vi "NI_controller.VI"(0 "Motion Settings":T1={"No Motion?"=FALSE, "Motion System"=enum."NI 735x", "Motion Bd ID"=1, "Motion Profile"="SMAC1", "# Axis"=1, "Reverse Z axis?"=TRUE, "SMAC Axis"=0, "scan pair"=enum."y-(x) scan", "RT fps"=6.0, "Steps per mm"=[1000, 1000, 1000, 1000], "Motor Parameters"={"velocity ct/s"=[10000.0, 10000.0, 10000.0, 50000.0], "accel ct/s^2"=[50000.0, 50000.0, 50000.0, 200000.0]}, "One Way Scan"=FALSE, "Reverse One Way Scan"=FALSE, "Global Position (mm)"=[], "Plane"=0, "Distance between\nscan lines (um)"=0.0, "Distance between\nscan planes (um)"=0.0, "number of scan planes"=1, "Total steps in line"=0, "Xtra plane\ndistance  (um)"=100, "Xtra planes "=1, "Add Axis"=FALSE, "overshoot cts"=200, "BKPT Shift"=0, "Scan Start Time (ms)"=0, "ESP VISA"="GPIB::1::INSTR", "3rd Axis"=1, "GL Ref Out"=refnum, "Galil Address"=""} {"3rd Axis" items=["x", "y", "z", "w"]; "Xtra planes" min=1; "Xtra plane\ndistance  (um)" min=0; "Distance between\nscan planes (um)" format="%.2f"; "Distance between\nscan lines (um)" format="%.2f"; "SMAC Axis" items=["None"=0, "Axis 1"=1, "Axis 2"=2, "Axis 3"=3, "Axis 4"=4, "Axis 5"=5, "Axis 6"=6, "Axis 7"=7, "Axis 8"=8, "Vector Space 1"=17, "Vector Space 2"=18, "Vector Space 3"=19, "Vector Space 4"=20]; "Motion Bd ID" min=1 max=32 step=1}, 4 "Initialize":bool=TRUE) -> (5 "Motion Settings Out":T1={"No Motion?"=FALSE, "Motion System"=enum."NI 735x", "Motion Bd ID"=1, "Motion Profile"="SMAC1", "# Axis"=1, "Reverse Z axis?"=TRUE, "SMAC Axis"=0, "scan pair"=enum."y-(x) scan", "RT fps"=6.0, "Steps per mm"=[1000, 1000, 1000, 1000], "Motor Parameters"={"velocity ct/s"=[10000.0, 10000.0, 10000.0, 50000.0], "accel ct/s^2"=[50000.0, 50000.0, 50000.0, 200000.0]}, "One Way Scan"=FALSE, "Reverse One Way Scan"=FALSE, "Global Position (mm)"=[], "Plane"=0, "Distance between\nscan lines (um)"=0.0, "Distance between\nscan planes (um)"=0.0, "number of scan planes"=1, "Total steps in line"=0, "Xtra plane\ndistance  (um)"=100, "Xtra planes "=1, "Add Axis"=FALSE, "overshoot cts"=200, "BKPT Shift"=0, "Scan Start Time (ms)"=0, "ESP VISA"="GPIB::1::INSTR", "3rd Axis"=1, "GL Ref Out"=refnum, "Galil Address"=""} {"3rd Axis" items=["x", "y", "z", "w"]; "Xtra planes" min=1; "Xtra plane\ndistance  (um)" min=0; "Distance between\nscan planes (um)" format="%.2f"; "Distance between\nscan lines (um)" format="%.2f"; "SMAC Axis" items=["None"=0, "Axis 1"=1, "Axis 2"=2, "Axis 3"=3, "Axis 4"=4, "Axis 5"=5, "Axis 6"=6, "Axis 7"=7, "Axis 8"=8, "Vector Space 1"=17, "Vector Space 2"=18, "Vector Space 3"=19, "Vector Space 4"=20]; "Motion Bd ID" min=1 max=32 step=1}, 6 "error out":errorcluster)   [LabVIEW 2022 SP3]
uses:
  -NI_MotionRoutines/MotionParameters.ctl
  -NI_MotionRoutines/MotionSys.ctl
  -MotionRoutines/ScanAxis.ctl
  -MotionRoutines/3rdAxis.ctl
  <vilib>/Motion/FlexMotion/CustomControls/CustomControls.llb/AxisOrVectorSpace To Configure.flx
  <vilib>/Motion/FlexMotion/FunctionsVIs/StartStopMotion.llb/Start Motion (8 axes).flx
  <vilib>/Motion/FlexMotion/FunctionsVIs/StartStopMotion.llb/Stop Motion (8 axes).flx
  -MotionRoutines/MotionGlobals.vi
  <vilib>/Motion/FlexMotion/FunctionsVIs/Trajectory.llb/Load Acceleration/Deceleration.flx
  <vilib>/event_ctls.llb/eventvkey.ctl
  <vilib>/Motion/FlexMotion/CustomControls/CustomControls.llb/Axis # (8 axes).flx
panel:
  in  "Cent All":bool
  in  "Position (mm) (Abs)":dbl format="%.3f"
  in  "Axis Tune":enum32{"Axis 1", "Axis 2", "Axis 3", "Axis 4"}(radio)
  in  "Inc. Step\nSize (mm)":dbl=0.5
  out "Found Center":bool
  in  "Cent X":bool
  in  "Cent Y":bool
  in  "Cent Z":bool
  in  "Abs W Pos (mm)":dbl format="%.3f"
  in  "Abs Z Pos (mm)":dbl format="%.3f"
  in  "Abs Y Pos (mm)":dbl format="%.3f"
  in  "Abs X Pos (mm)":dbl format="%.3f"
  in  "Def Abs":bool
  in  "Select V&A":bool
  in  "Slave Axis":u16(ring)=2 items=["Axis 1"=1, "Axis 2"=2, "Axis 3"=3, "Axis 4"=4]
  in  "Master Axis":u16(ring)=1 items=["Axis 1"=1, "Axis 2"=2, "Axis 3"=3, "Axis 4"=4]
  in  "Enable Gearing":bool
  out "Angle":dbl=45.000038009906035
  in  "Ratio Denom":u16=1 min=1 max=32767
  in  "Ratio Num":i16 min=0
  in  "Cent W":bool
  in  "W Position (mm)":dbl format="%.3f"
  in  "FineMi4":bool
  in  "FinePl4":bool
  in  "Rst4":bool
  in  "Ax4Plus":bool
  in  "Ax4Minus":bool
  in  "Z Position (mm)":dbl format="%.3f"
  in  "FineMi3":bool
  in  "FinePl3":bool
  in  "Rst3":bool
  in  "Ax3Plus":bool
  in  "Ax3Minus":bool
  in  "Y Position (mm)":dbl format="%.3f"
  in  "FineMi2":bool
  in  "FinePl2":bool
  in  "Rst2":bool
  in  "Ax2Plus":bool
  in  "Ax2Minus":bool
  in  "X Position (mm)":dbl format="%.3f"
  in  "stop":bool
  in  "FineMi1":bool
  in  "FinePl1":bool
  in  "Rst1":bool
  in  "Ax1Plus":bool
  in  "Ax1Minus":bool
  # "Units are in mm. \"Rst\" zeros the position. Blue circles move 1 cm for linear."
  # "Redefine\nAbs Position"
  # "Be very careful with this mode it is not fully programmed"
  # "X Axis (mm)"
  # "Y Axis  (mm)"
  # "Z Axis (mm)"
  # "LinInd (mm)"
  # "1-D and 2-D B scan settings"
  # "1-D and 2-D B scan settings"
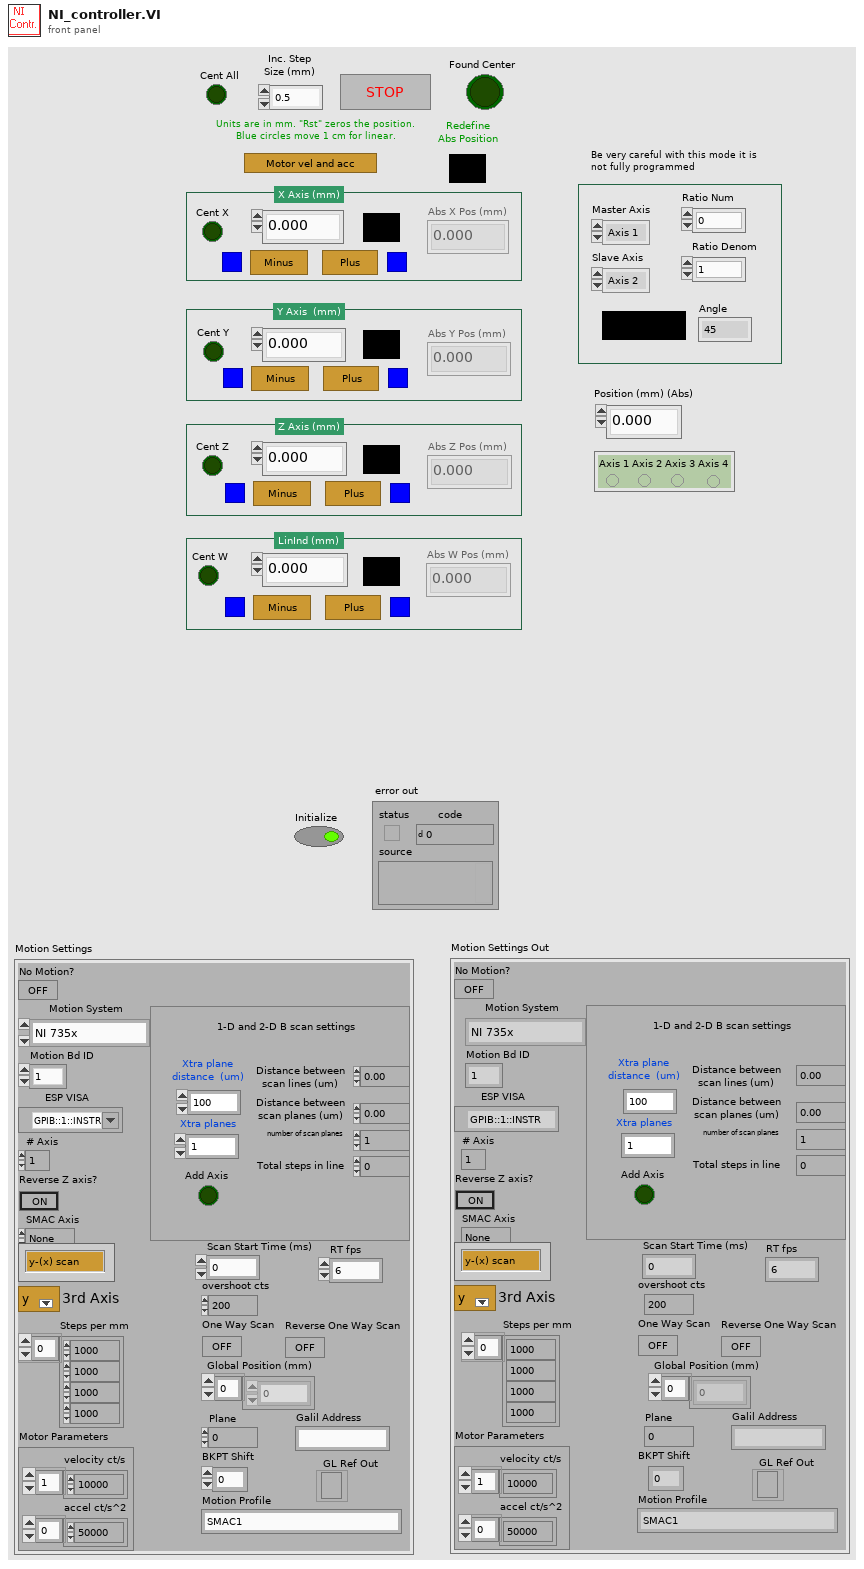
[diagram p1: front panel]
types:
  T1 = typedef "MotionParameters.ctl" = cluster{"No Motion?":bool, "Motion System":T2, "Motion Bd ID":u8, "Motion Profile":string, "# Axis":i8, "Reverse Z axis?":bool, "SMAC Axis":u16, "scan pair":T3, "RT fps":sgl, "Steps per mm":i32[], "Motor Parameters":cluster{"velocity ct/s":dbl[], "accel ct/s^2":dbl[]}, "One Way Scan":bool, "Reverse One Way Scan":bool, "Global Position (mm)":dbl[], "Plane":i32, "Distance between\nscan lines (um)":sgl, "Distance between\nscan planes (um)":sgl, "number of scan planes":i32, "Total steps in line":i32, "Xtra plane\ndistance  (um)":i32, "Xtra planes ":i32, "Add Axis":bool, "overshoot cts":i32, "BKPT Shift":i32, "Scan Start Time (ms)":u32, "ESP VISA":refnum<visa-resource-name>, "3rd Axis":T4, "GL Ref Out":refnum<k7>, "Galil Address":string}
  T2 = typedef "MotionSys.ctl" = enum16{"MM3000", "NI 735x", "Newport ESP", "No Motion Card", "Galil"}
  T3 = typedef "ScanAxis.ctl" = enum16{"y-(x) scan", "x-(y) scan", "z-(x) scan", "z-(y) scan", "y-(z) scan", "x-(z) scan", "w-(x) scan", "w-(y) scan", "w-(z) scan", "x-(w) scan", "y-(w) scan", "z-(w) scan"}
  T4 = typedef "3rdAxis.ctl" = u16
  T5 = enum16{"Absolute Position", "Relative Position", "Velocity", "Relative to Cap Pos", "Modulus Position", "Absolute Contouring", "Relative Contouring"}
  T6 = enum16{"Home", "Index", "Center", "Forward Limit", "Reverse Limit", "Run Sequence"}
  T7 = typedef "Axis # (8 axes).flx" = cluster{"1":bool, "2":bool, "3":bool, "4":bool, "5":bool, "6":bool, "7":bool, "8":bool}
  T8 = enum8{"Enabled", "Disabled", "Disabled and Grayed Out"}
  T9 = typedef "Bd Id Out" = u8
  T10 = typedef "location.ctl" = enum16{"Automatic", "WCM Main", "Hawaii", "Columbia MM3000", "Columbia  NI System", "NYU", "RRI 2", "UHI Allen", "CUMC RT", "Chiba", "Stony Brook", "WCM Microscopy", "WCM Aeoretch", "WCM Optics Lab", "WCM Main 2Axis", "WCM Rotation", "WCM SAM SMAC", "SERI GP"}
  T11 = typedef "AxisOrVectorSpace To Configure.flx" = u16
  T12 = cluster{"Steps per mm[0]":i32, "Steps per mm[1]":i32, "Steps per mm[2]":i32, "Steps per mm[3]":i32}
  T13 = typedef "Resource Out (Enum).flx" = u16
  T14 = typedef "eventvkey.ctl" = enum16{"ASCII", "Enter", "Return", "Shift", "Ctrl", "Alt", "Cmd", "Opt", "Caps", "NumLock", "Clear", "Break", "Up", "Down", "Left", "Right", "Insert", "Delete", "Home", "End", "PageUp", "PageDown", "Escape", "Help", "Pause", "ScrollLock", "F1", "F2", "F3", "F4", "F5", "F6", "F7", "F8", "F9", "F10", "F11", "F12", "F13", "F14", "F15", "F16", "F17", "F18", "F19", "F20", "F21", "F22", "F23", "F24", "Play", "VolumeUp", "VolumeDown", "Mute", "Two Byte Char"}
  T15 = cluster{"Shift":bool, "Ctrl":bool, "Alt":bool, "Cmd":bool, "Opt":bool}
  T16 = typedef "AxisOrVectorSpaceControl To Control.flx" = u16
  T17 = cluster{"Axis/VS Map (Disabled)[0]":bool, "Axis/VS Map (Disabled)[1]":bool, "Axis/VS Map (Disabled)[2]":bool, "Axis/VS Map (Disabled)[3]":bool, "Axis/VS Map (Disabled)[4]":bool, "Axis/VS Map (Disabled)[5]":bool, "Axis/VS Map (Disabled)[6]":bool, "Axis/VS Map (Disabled)[7]":bool, "Axis/VS Map (Disabled)[8]":bool}
  T18 = cluster{"Axis/VS Map (Disabled)[1]":bool, "Axis/VS Map (Disabled)[2]":bool, "Axis/VS Map (Disabled)[3]":bool, "Axis/VS Map (Disabled)[4]":bool, "Axis/VS Map (Disabled)[5]":bool, "Axis/VS Map (Disabled)[6]":bool, "Axis/VS Map (Disabled)[7]":bool, "Axis/VS Map (Disabled)[8]":bool}
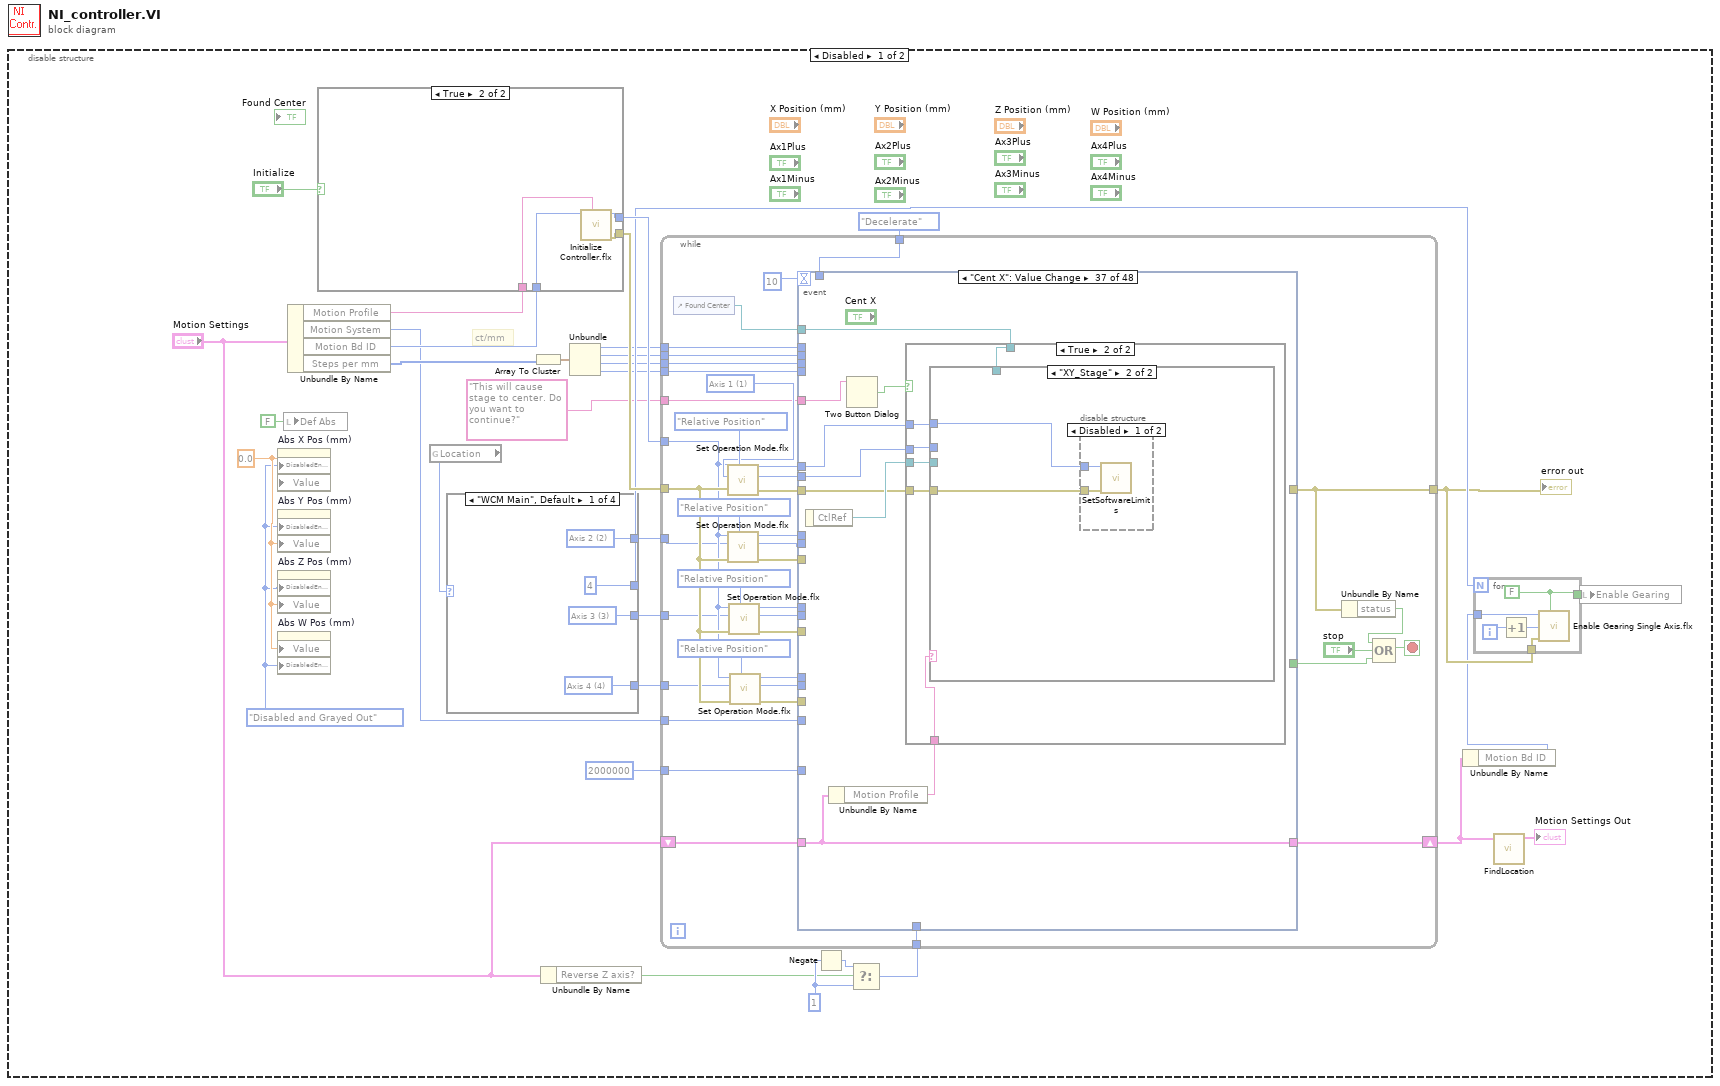
[diagram p0: block diagram]
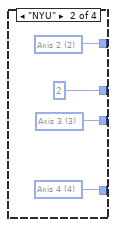
[diagram p2: hidden frame]
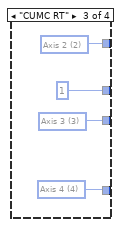
[diagram p3: hidden frame]
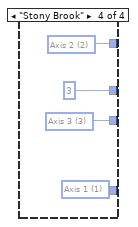
[diagram p4: hidden frame]
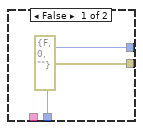
[diagram p5: hidden frame]
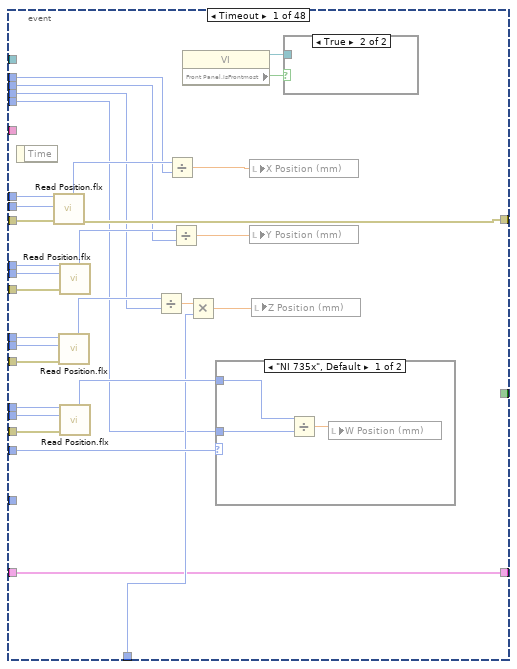
[diagram p6: hidden frame]
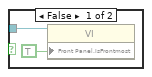
[diagram p7: hidden frame]
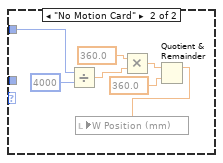
[diagram p8: hidden frame]
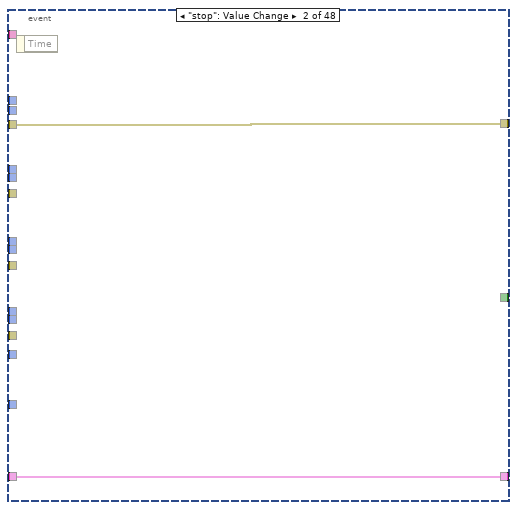
[diagram p9: hidden frame]
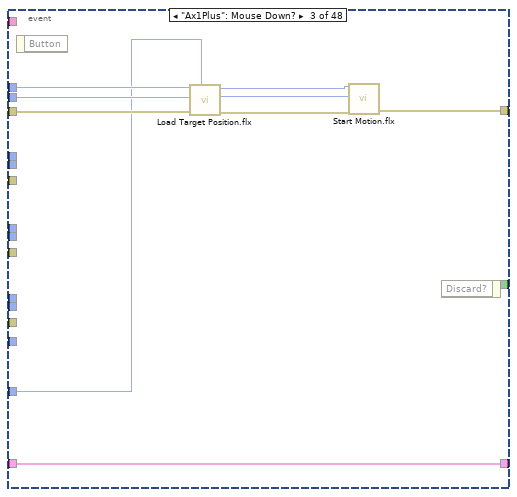
[diagram p10: hidden frame]
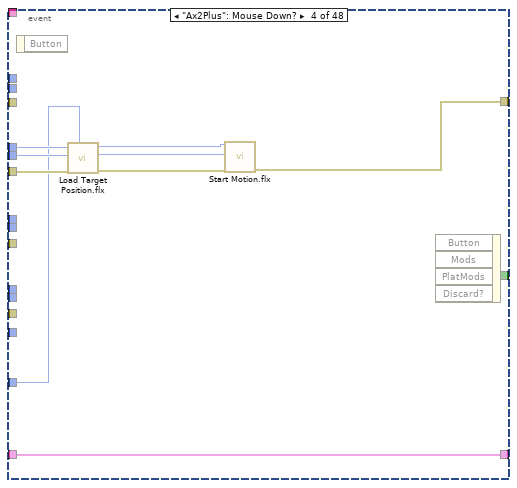
[diagram p11: hidden frame]
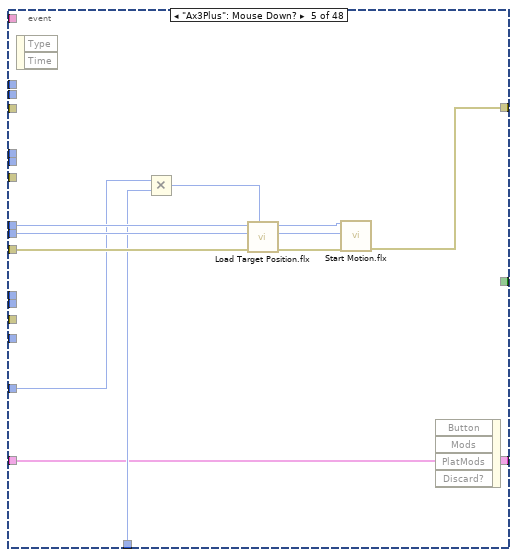
[diagram p12: hidden frame]
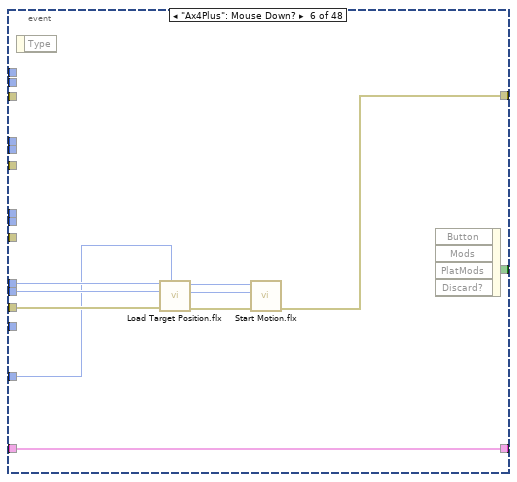
[diagram p13: hidden frame]
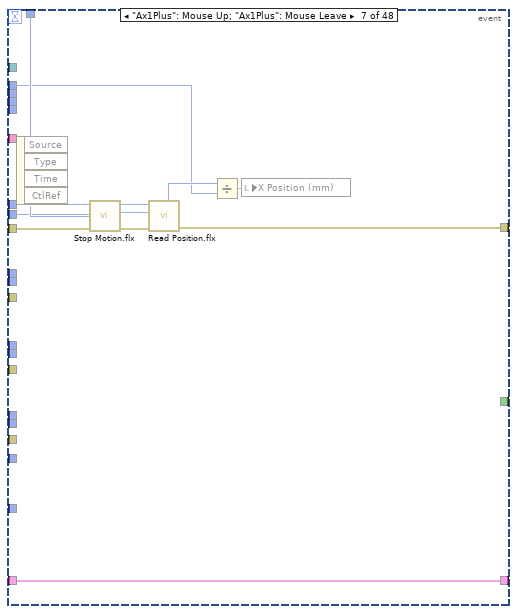
[diagram p14: hidden frame]
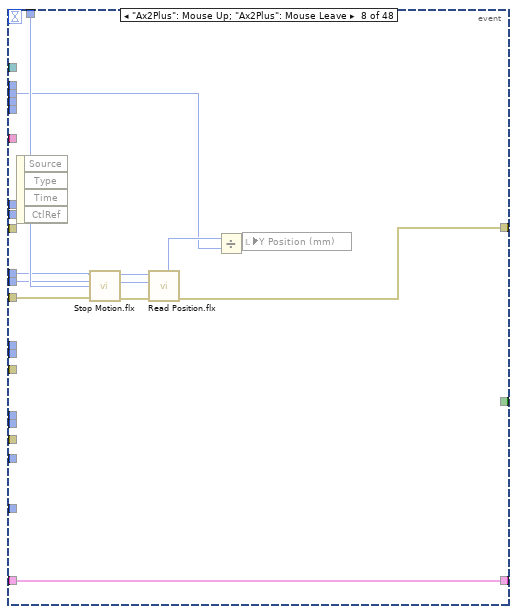
[diagram p15: hidden frame]
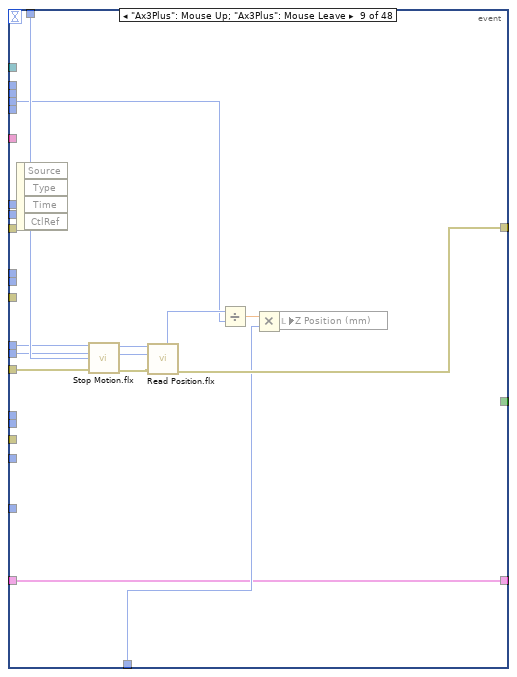
[diagram p16: hidden frame]
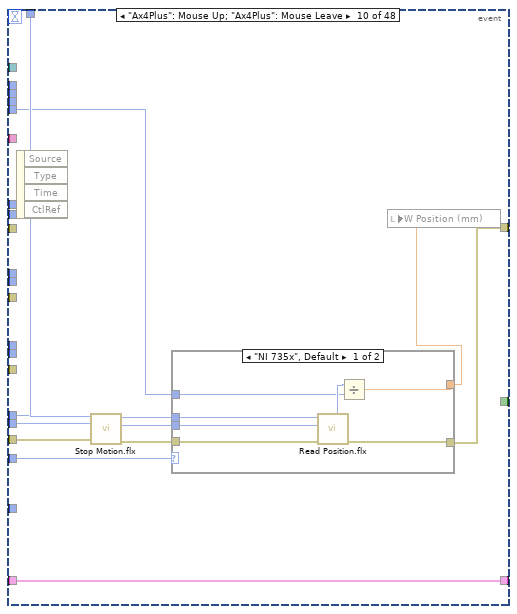
[diagram p17: hidden frame]
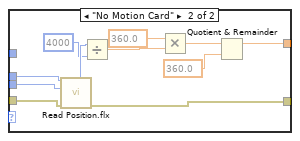
[diagram p18: hidden frame]
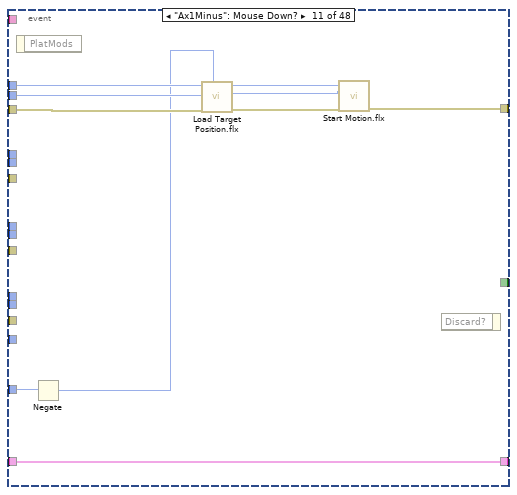
[diagram p19: hidden frame]
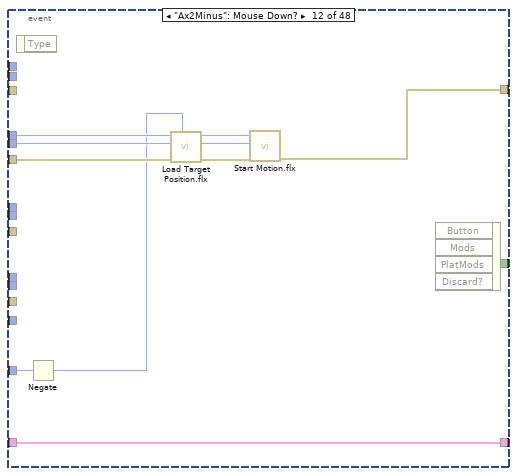
[diagram p20: hidden frame]
diagram:
  n1 = disable-structure shown="Disabled" {
    frame Disabled {
      w5 = T8."Disabled and Grayed Out" ("Disabled")
      w14 = 0.0 ("Abs X Pos (mm)")
      w28 = 1
      # "ct/mm"
      n2 = property on="Abs X Pos (mm)" class="DigNum (strict)"("DisabledEnum"=w5, "Value"=w14) -> ()  [unwired: 2 in, 2 out]
      n3 = property on="Abs Y Pos (mm)" class="DigNum (strict)"("DisabledEnum"=w5, "Value"=w14) -> ()  [unwired: 2 in, 2 out]
      n4 = property on="Abs Z Pos (mm)" class="DigNum (strict)"("DisabledEnum"=w5, "Value"=w14) -> ()  [unwired: 2 in, 2 out]
      n5 = property on="Abs W Pos (mm)" class="DigNum (strict)"("Value"=w14, "DisabledEnum"=w5) -> ()  [unwired: 2 in, 2 out]
      n6 = local write "Def Abs"(FALSE ("Visible")) -> ()
      n7 = Unbundle By Name("Motion Settings") -> ("Motion Profile"=w2:string, "Motion System"=w7:T2, "Motion Bd ID"=w13:u8, "Steps per mm"=w11:i32[])
      n8 = case shown="True" "Initialize" {
        tunnel: [w56 w60] -> w33
        tunnel: [errorcluster {"status"=FALSE, "code"=0, "source"=""} ("error out") w59] -> w32
        tunnel: w13 -> [w56 w58]
        tunnel: w2 -> [_ w57]
        frame False {
        }
        frame True {
          n9 = call <vilib>:"Initialize Controller.flx"("Settings Name"=w57, "Board ID"=w58) -> ("error out"=w59:errorcluster, "Bd ID Out"=w60:T9)  [unwired: 1 in, 5 out]
        }
      }
      n10 = global read "MotionGlobals.vi" "Location"() -> (w22:T10)
      n11 = case shown="\"WCM Main\", Default" w22 {
        tunnel: [w37 w40 w44 w48] -> w25
        tunnel: [w36 w41 w45 w49] -> w24
        tunnel: [4 2 1 3] -> w23
        tunnel: [w34 w38 w42 w46] -> w21
        frame "WCM Main", Default {
          w34 = T11 2 items=["Axis Control"=0, "Axis 1"=1, "Axis 2"=2, "Axis 3"=3, "Axis 4"=4, "Axis 5"=5, "Axis 6"=6, "Axis 7"=7, "Axis 8"=8, "Vector Space Control"=16, "Vector Space 1"=17, "Vector Space 2"=18, "Vector Space 3"=19, "Vector Space 4"=20] ("Axis or Vector Space")
          w37 = T11 4 items=["Axis Control"=0, "Axis 1"=1, "Axis 2"=2, "Axis 3"=3, "Axis 4"=4, "Axis 5"=5, "Axis 6"=6, "Axis 7"=7, "Axis 8"=8, "Vector Space Control"=16, "Vector Space 1"=17, "Vector Space 2"=18, "Vector Space 3"=19, "Vector Space 4"=20] ("Axis or Vector Space")
          w36 = T11 3 items=["Axis Control"=0, "Axis 1"=1, "Axis 2"=2, "Axis 3"=3, "Axis 4"=4, "Axis 5"=5, "Axis 6"=6, "Axis 7"=7, "Axis 8"=8, "Vector Space Control"=16, "Vector Space 1"=17, "Vector Space 2"=18, "Vector Space 3"=19, "Vector Space 4"=20] ("Axis or Vector Space")
        }
        frame "NYU" {
          w38 = T11 2 items=["Axis Control"=0, "Axis 1"=1, "Axis 2"=2, "Axis 3"=3, "Axis 4"=4, "Axis 5"=5, "Axis 6"=6, "Axis 7"=7, "Axis 8"=8, "Vector Space Control"=16, "Vector Space 1"=17, "Vector Space 2"=18, "Vector Space 3"=19, "Vector Space 4"=20] ("Axis or Vector Space")
          w40 = T11 4 items=["Axis Control"=0, "Axis 1"=1, "Axis 2"=2, "Axis 3"=3, "Axis 4"=4, "Axis 5"=5, "Axis 6"=6, "Axis 7"=7, "Axis 8"=8, "Vector Space Control"=16, "Vector Space 1"=17, "Vector Space 2"=18, "Vector Space 3"=19, "Vector Space 4"=20] ("Axis or Vector Space")
          w41 = T11 3 items=["Axis Control"=0, "Axis 1"=1, "Axis 2"=2, "Axis 3"=3, "Axis 4"=4, "Axis 5"=5, "Axis 6"=6, "Axis 7"=7, "Axis 8"=8, "Vector Space Control"=16, "Vector Space 1"=17, "Vector Space 2"=18, "Vector Space 3"=19, "Vector Space 4"=20] ("Axis or Vector Space")
        }
        frame "CUMC RT" {
          w42 = T11 2 items=["Axis Control"=0, "Axis 1"=1, "Axis 2"=2, "Axis 3"=3, "Axis 4"=4, "Axis 5"=5, "Axis 6"=6, "Axis 7"=7, "Axis 8"=8, "Vector Space Control"=16, "Vector Space 1"=17, "Vector Space 2"=18, "Vector Space 3"=19, "Vector Space 4"=20] ("Axis or Vector Space")
          w44 = T11 4 items=["Axis Control"=0, "Axis 1"=1, "Axis 2"=2, "Axis 3"=3, "Axis 4"=4, "Axis 5"=5, "Axis 6"=6, "Axis 7"=7, "Axis 8"=8, "Vector Space Control"=16, "Vector Space 1"=17, "Vector Space 2"=18, "Vector Space 3"=19, "Vector Space 4"=20] ("Axis or Vector Space")
          w45 = T11 3 items=["Axis Control"=0, "Axis 1"=1, "Axis 2"=2, "Axis 3"=3, "Axis 4"=4, "Axis 5"=5, "Axis 6"=6, "Axis 7"=7, "Axis 8"=8, "Vector Space Control"=16, "Vector Space 1"=17, "Vector Space 2"=18, "Vector Space 3"=19, "Vector Space 4"=20] ("Axis or Vector Space")
        }
        frame "Stony Brook" {
          w46 = T11 2 items=["Axis Control"=0, "Axis 1"=1, "Axis 2"=2, "Axis 3"=3, "Axis 4"=4, "Axis 5"=5, "Axis 6"=6, "Axis 7"=7, "Axis 8"=8, "Vector Space Control"=16, "Vector Space 1"=17, "Vector Space 2"=18, "Vector Space 3"=19, "Vector Space 4"=20] ("Axis or Vector Space")
          w48 = T11 1 items=["Axis Control"=0, "Axis 1"=1, "Axis 2"=2, "Axis 3"=3, "Axis 4"=4, "Axis 5"=5, "Axis 6"=6, "Axis 7"=7, "Axis 8"=8, "Vector Space Control"=16, "Vector Space 1"=17, "Vector Space 2"=18, "Vector Space 3"=19, "Vector Space 4"=20] ("Axis or Vector Space")
          w49 = T11 3 items=["Axis Control"=0, "Axis 1"=1, "Axis 2"=2, "Axis 3"=3, "Axis 4"=4, "Axis 5"=5, "Axis 6"=6, "Axis 7"=7, "Axis 8"=8, "Vector Space Control"=16, "Vector Space 1"=17, "Vector Space 2"=18, "Vector Space 3"=19, "Vector Space 4"=20] ("Axis or Vector Space")
        }
      }
      n12 = Array To Cluster(array=w11) -> (cluster=w20:T12)
      n13 = Unbundle By Name("Motion Settings") -> ("Reverse Z axis?"=w12:bool)
      n14 = Unbundle(w20) -> ("Steps per mm[0]"=w19:i32, "Steps per mm[1]"=w18:i32, "Steps per mm[2]"=w17:i32, "Steps per mm[3]"=w16:i32)
      n15 = Negate(x=w28) -> (-x=w30:i32)
      n16 = Select(t=w30, s=w12, f=w28) -> (s? t:f=w29:i32)
      n17 = while {
        tunnel: [w76] -> w9
        tunnel: w32 -> [w89]
        tunnel: w33 -> [w81]
        tunnel: w29 -> [w78]
        tunnel: w7 -> [w77]
        tunnel: 2000000 -> [w75]
        tunnel: enum16{"Decelerate", "Halt", "Kill"}."Decelerate" ("Stop Type (Decel)") -> [w74]
        tunnel: w25 -> [w73]
        tunnel: w24 -> [w72]
        tunnel: w21 -> [w71]
        tunnel: w19 -> [w70]
        tunnel: w18 -> [w69]
        tunnel: w17 -> [w68]
        tunnel: w16 -> [w67]
        shift-right: [w65] -> w4
        shift-left: "Motion Settings" -> [w66]
        tunnel: "This will cause stage to center. Do you want to continue?" ("message") -> [w61]
        stop <- w99 stop-if-true
        w94 = T11 1 items=["Axis Control"=0, "Axis 1"=1, "Axis 2"=2, "Axis 3"=3, "Axis 4"=4, "Axis 5"=5, "Axis 6"=6, "Axis 7"=7, "Axis 8"=8, "Vector Space Control"=16, "Vector Space 1"=17, "Vector Space 2"=18, "Vector Space 3"=19, "Vector Space 4"=20] ("Axis or Vector Space")
        n18 = control-ref of="Found Center"() -> (w63:refnum<vi>)
        n19 = call <vilib>:"Set Operation Mode.flx"("Position Mode (Absolute)"=T5."Relative Position", "error in (no error)"=w89, "Axis or Vector Space"=w94, "Board ID"=w81) -> ("error out"=w96:errorcluster, "Resource Output"=w93:T13, "Bd ID Out"=w97:T9)  [unwired: 2 out]
        n20 = call <vilib>:"Set Operation Mode.flx"("Position Mode (Absolute)"=T5."Relative Position", "error in (no error)"=w89, "Axis or Vector Space"=w71, "Board ID"=w81) -> ("error out"=w88:errorcluster, "Resource Output"=w80:T13, "Bd ID Out"=w79:T9)  [unwired: 2 out]
        n21 = call <vilib>:"Set Operation Mode.flx"("Position Mode (Absolute)"=T5."Relative Position", "error in (no error)"=w89, "Axis or Vector Space"=w72, "Board ID"=w81) -> ("error out"=w85:errorcluster, "Resource Output"=w86:T13, "Bd ID Out"=w87:T9)  [unwired: 2 out]
        n22 = call <vilib>:"Set Operation Mode.flx"("Position Mode (Absolute)"=T5."Relative Position", "error in (no error)"=w89, "Axis or Vector Space"=w73, "Board ID"=w81) -> ("error out"=w82:errorcluster, "Resource Output"=w83:T13, "Bd ID Out"=w84:T9)  [unwired: 2 out]
        n23 = event shown="[36] \"Cent X\": Value Change" {
          selector: _ -> [_ _ _ _ _ _ _ _ _ _ _ _ _ _ _ _ _ _ _ _ _ _ _ _ _ _ _ _ _ _ _ _ _ _ _ _ _ _ _ _ _ _ _ _ _ _ _ _]
          dyn-events: _ -> [_ _ _ _ _ _ _ _ _ _ _ _ _ _ _ _ _ _ _ _ _ _ _ _ _ _ _ _ _ _ _ _ _ _ _ _ _ _ _ _ _ _ _ _ _ _ _ _]
          timeout: 10 -> [_ _ _ _ _ _ _ _ _ _ _ _ _ _ _ _ _ _ _ _ _ _ _ _ _ _ _ _ _ _ _ _ _ _ _ _ _ _ _ _ _ _ _ _ _ _ _ _]
          tunnel: w97 -> [w130 _ w153 _ _ _ w194 _ _ _ w260 _ _ _ w303 _ _ _ w366 _ _ _ w391 _ _ _ w447 _ _ _ w513 _ _ _ _ _ w646 _ _ _ _ _ _ _ w824 _ _ _]
          tunnel: w96 -> [w129 w144 w151 _ _ _ w193 _ _ _ w258 _ _ _ w302 _ _ _ w365 _ _ _ w390 _ _ _ w446 _ _ _ w512 _ _ _ _ _ w650 _ _ _ _ _ _ _ _ _ _ _]
          tunnel: w74 -> [_ _ _ _ _ _ w192 w202 w216 w232 _ _ _ _ w304 w312 w326 w339 _ _ _ _ _ _ _ _ _ _ _ _ _ _ _ _ _ _ _ _ _ _ _ _ _ _ _ _ _ _]
          tunnel: w93 -> [w106 _ w152 _ _ _ w186 _ _ _ w259 _ _ _ w295 _ _ _ w364 _ _ _ w388 _ _ _ w444 _ _ _ w499 _ _ _ _ _ w645 _ _ _ _ _ _ _ w823 _ _ _]
          tunnel: w79 -> [w125 _ _ w159 _ _ _ w201 _ _ _ w267 _ _ _ w311 _ _ _ w372 _ _ _ w401 _ _ _ w457 _ _ _ w520 _ _ _ _ _ w688 _ _ _ w800 w811 _ _ w830 _ _]
          tunnel: w80 -> [w115 _ _ w158 _ _ _ w200 _ _ _ w266 _ _ _ w310 _ _ _ w371 _ _ _ w400 _ _ _ w456 _ _ _ w518 _ _ _ _ _ w687 _ _ _ _ _ _ _ w829 _ _]
          tunnel: w88 -> [w124 _ _ w157 _ _ _ w199 _ _ _ w265 _ _ _ w309 _ _ _ w370 _ _ _ w399 _ _ _ w455 _ _ _ w519 _ _ _ _ _ w685 _ _ _ _ _ _ _ _ _ _]
          tunnel: w87 -> [w123 _ _ _ w170 _ _ _ w215 _ _ _ w279 _ _ _ w325 _ _ _ w378 _ _ _ w413 _ _ _ w469 _ _ _ w538 _ _ _ _ _ w721 _ _ _ _ _ _ _ w838 _]
          tunnel: w86 -> [w122 _ _ _ w169 _ _ _ w214 _ _ _ w278 _ _ _ w324 _ _ _ w377 _ _ _ w412 _ _ _ w468 _ _ _ w537 _ _ _ _ _ w720 _ _ _ _ _ _ _ w837 _]
          tunnel: w85 -> [w121 _ _ _ w168 _ _ _ w213 _ _ _ w277 _ _ _ w323 _ _ _ w376 _ _ _ w411 _ _ _ w467 _ _ _ w536 _ _ _ _ _ w718 _ _ _ _ _ _ _ _ _]
          tunnel: w84 -> [w120 _ _ _ _ w179 _ _ _ w231 _ _ _ w289 _ _ _ w338 _ _ _ w384 _ _ _ w424 _ _ _ w480 _ _ _ w557 w588 _ _ _ _ w757 w763 _ _ _ _ _ _ w844]
          tunnel: w83 -> [w119 _ _ _ _ w178 _ _ _ w230 _ _ _ w288 _ _ _ w337 _ _ _ w383 _ _ _ w423 _ _ _ w479 _ _ _ w556 _ _ _ _ _ w756 _ _ _ _ _ _ _ w843]
          tunnel: w82 -> [w118 _ _ _ _ w177 _ _ _ w229 _ _ _ w287 _ _ _ w336 _ _ _ w382 _ _ _ w422 _ _ _ w478 _ _ _ w555 w589 _ _ _ _ w747 w762 _ _ _ _ _ _ _]
          tunnel: [w112 w144 w147 w156 w165 w176 w185 w197 w212 w223 w254 w264 w273 w286 w296 w307 w322 w333 w362 w368 w374 _ w389 w398 w408 w421 w445 w454 w464 w477 w500 w516 w534 w552 w586 _ _ _ _ _ _ _ _ _ _ _ _ _] -> w76
          tunnel: [_ _ _ _ _ _ _ _ _ _ _ _ _ _ _ _ _ _ _ _ _ w381 _ _ _ _ _ _ _ _ _ _ _ _ _ _ _ _ _ _ _ _ _ _ _ _ _ _] -> _
          tunnel: w78 -> [w109 _ _ _ w167 _ _ _ w209 _ _ _ w276 _ _ _ w319 _ _ _ _ _ _ _ w410 _ _ _ w466 _ _ _ w533 _ _ _ _ _ _ _ _ _ _ _ _ _ w833 _]
          tunnel: w77 -> [w113 _ _ _ _ _ _ _ _ w224 _ _ _ _ _ _ _ w334 _ _ _ _ _ _ _ w420 _ _ _ w476 _ _ _ w551 _ _ _ _ _ _ _ _ _ _ _ _ _ _]
          tunnel: w75 -> [_ _ w146 w155 w164 w175 _ _ _ _ w253 w263 w272 w285 _ _ _ _ _ _ _ _ _ _ _ _ _ _ _ _ _ _ _ _ _ _ _ _ _ _ _ _ _ _ _ _ _ _]
          tunnel: w70 -> [w105 _ _ _ _ _ w184 _ _ _ _ _ _ _ w294 _ _ _ _ _ _ _ w386 _ _ _ w442 _ _ _ w498 _ _ _ _ _ _ _ _ _ _ _ _ _ w822 _ _ _]
          tunnel: w69 -> [w104 _ _ _ _ _ _ w196 _ _ _ _ _ _ _ w306 _ _ _ _ _ _ _ w397 _ _ _ w453 _ _ _ w515 _ _ _ _ _ _ _ _ _ _ _ _ _ w828 _ _]
          tunnel: w68 -> [w103 _ _ _ _ _ _ _ w208 _ _ _ _ _ _ _ w318 _ _ _ _ _ _ _ w407 _ _ _ w463 _ _ _ w532 _ _ _ _ _ _ _ _ _ _ _ _ _ w836 _]
          tunnel: w67 -> [w102 _ _ _ _ _ _ _ _ w222 _ _ _ _ _ _ _ w332 _ _ _ _ _ _ _ w419 _ _ _ w475 _ _ _ w550 _ _ _ _ _ _ _ _ _ _ _ _ _ w842]
          tunnel: w66 -> [w101 w143 w145 w154 w163 w174 w183 w195 w207 w221 w251 w261 w271 w283 w293 w305 w317 w331 w361 w367 w373 w379 w385 w395 w405 w417 w441 w451 w461 w473 w497 w514 w531 w549 w583 w617 w644 w680 w722 w751 w759 w798 w810 w816 w819 w825 w831 w839]
          tunnel: [w101 w143 w145 w154 w163 w174 w183 w195 w207 w221 w251 w261 w271 w283 w293 w305 w317 w331 w361 w367 w373 w379 w385 w395 w405 w417 w441 w451 w461 w473 w497 w514 w531 w549 w582 w617 w644 w680 w722 w751 w759 w798 w810 w816 w819 w825 w831 w839] -> w65
          tunnel: w63 -> [_ _ _ _ _ _ _ _ _ _ _ _ _ _ _ _ _ _ _ _ _ _ _ _ _ _ _ _ _ _ _ _ _ _ _ _ w649 w683 w717 w743 w760 _ _ _ _ _ _ _]
          tunnel: [_ _ _ _ _ _ _ _ _ _ _ _ _ _ _ _ _ _ _ _ _ _ _ _ _ _ _ _ _ _ _ _ _ _ _ w615 _ _ _ _ _ _ _ _ _ _ _ _] -> w62
          tunnel: w61 -> [_ _ _ _ _ _ _ _ _ _ _ _ _ _ _ _ _ _ _ _ _ _ _ _ _ _ _ _ _ _ _ _ _ _ _ _ w648 w682 w715 _ _ _ _ _ _ _ _ _]
          event Timeout {
            n24 = event-data() -> ()  [unwired: 2 out]
            n25 = call <vilib>:"Read Position.flx"("error in (no error)"=w129, "Axis"=w106, "Board ID"=w130) -> ("error out"=w112:errorcluster, "Position"=w128:i32)  [unwired: 5 out]
            n26 = call <vilib>:"Read Position.flx"("error in (no error)"=w121, "Axis"=w122, "Board ID"=w123) -> ("Position"=w111:i32)  [unwired: 6 out]
            n27 = call <vilib>:"Read Position.flx"("error in (no error)"=w124, "Axis"=w115, "Board ID"=w125) -> ("Position"=w126:i32)  [unwired: 6 out]
            n28 = call <vilib>:"Read Position.flx"("error in (no error)"=w118, "Axis"=w119, "Board ID"=w120) -> ("Position"=w114:i32)  [unwired: 6 out]
            n29 = Divide(x=w111, y=w103) -> (x/y=w110:dbl)
            n30 = Divide(x=w128, y=w105) -> (x/y=w127:dbl)
            n31 = Divide(x=w126, y=w104) -> (x/y=w117:dbl)
            n32 = property class="VI"() -> (reference out=w108:refnum<vi>, "Front Panel.IsFrontmost"=w107:bool)  [unwired: 2 in, 1 out]
            n33 = Multiply(x=w110, y=w109) -> (x*y=w116:dbl)
            n34 = case shown="\"NI 735x\", Default" w113 {
              tunnel: w114 -> [w135 w136]
              tunnel: w102 -> [w133 _]
              frame "NI 735x", Default {
                n35 = Divide(x=w135, y=w133) -> (x/y=w134:dbl)
                n36 = local write "W Position (mm)"(w134) -> ()
              }
              frame "No Motion Card" {
                n37 = Divide(x=w136, y=4000) -> (x/y=w141:dbl)
                n38 = Multiply(x=360.0, y=w141) -> (x*y=w138:dbl)
                n39 = Quotient & Remainder(x=w138, y=360.0) -> (x-y*floor(x/y)=w137:dbl)  [unwired: 1 out]
                n40 = local write "W Position (mm)"(w137) -> ()
              }
            }
            n41 = local write "X Position (mm)"(w127) -> ()
            n42 = local write "Y Position (mm)"(w117) -> ()
            n43 = local write "Z Position (mm)"(w116) -> ()
            n44 = case shown="True" w107 {
              tunnel: w108 -> [w132 _]
              frame False {
                n45 = property class="VI"(reference=w132, "Front Panel.IsFrontmost"=TRUE) -> ()  [unwired: 1 in, 2 out]
              }
              frame True {
              }
            }
          }
          event "stop": Value Change {
            n46 = event-data() -> ()  [unwired: 2 out]
          }
          event "Ax1Plus": Mouse Down? {
            n47 = event-data() -> ()  [unwired: 2 out]
            n48 = call <vilib>:"Load Target Position.flx"("Target Position (0)"=w146, "error in (no error)"=w151, "Axis"=w152, "Board ID"=w153) -> ("error out"=w150:errorcluster, "Resource Output"=w149:T13, "Bd ID Out"=w148:T9)  [unwired: 3 out]
            n49 = call-poly <vilib>:"Start Motion.flx"("error in (no error)"=w150, "Axis or Vector Space"=w149, "Board ID"=w148) -> ("error out"=w147:errorcluster)  [unwired: 1 in, 4 out]
            n50 = event-data() -> ()  [unwired: 1 in, 2 out]
          }
          event "Ax2Plus": Mouse Down? {
            n51 = event-data() -> ()  [unwired: 2 out]
            n52 = call <vilib>:"Load Target Position.flx"("Target Position (0)"=w155, "error in (no error)"=w157, "Axis"=w158, "Board ID"=w159) -> ("error out"=w162:errorcluster, "Resource Output"=w161:T13, "Bd ID Out"=w160:T9)  [unwired: 3 out]
            n53 = call-poly <vilib>:"Start Motion.flx"("error in (no error)"=w162, "Axis or Vector Space"=w161, "Board ID"=w160) -> ("error out"=w156:errorcluster)  [unwired: 1 in, 4 out]
            n54 = event-data() -> ()  [unwired: 1 in, 5 out]
          }
          event "Ax3Plus": Mouse Down? {
            n55 = event-data() -> ()  [unwired: 3 out]
            n56 = Multiply(x=w164, y=w167) -> (x*y=w166:i32)
            n57 = call <vilib>:"Load Target Position.flx"("Target Position (0)"=w166, "error in (no error)"=w168, "Axis"=w169, "Board ID"=w170) -> ("error out"=w173:errorcluster, "Resource Output"=w172:T13, "Bd ID Out"=w171:T9)  [unwired: 3 out]
            n58 = call-poly <vilib>:"Start Motion.flx"("error in (no error)"=w173, "Axis or Vector Space"=w172, "Board ID"=w171) -> ("error out"=w165:errorcluster)  [unwired: 1 in, 4 out]
            n59 = event-data() -> ()  [unwired: 1 in, 5 out]
          }
          event "Ax4Plus": Mouse Down? {
            n60 = event-data() -> ()  [unwired: 2 out]
            n61 = call <vilib>:"Load Target Position.flx"("Target Position (0)"=w175, "error in (no error)"=w177, "Axis"=w178, "Board ID"=w179) -> ("error out"=w182:errorcluster, "Resource Output"=w181:T13, "Bd ID Out"=w180:T9)  [unwired: 3 out]
            n62 = call-poly <vilib>:"Start Motion.flx"("error in (no error)"=w182, "Axis or Vector Space"=w181, "Board ID"=w180) -> ("error out"=w176:errorcluster)  [unwired: 1 in, 4 out]
            n63 = event-data() -> ()  [unwired: 1 in, 5 out]
          }
          event "Ax1Plus": Mouse Up; "Ax1Plus": Mouse Leave {
            n64 = event-data() -> ()  [unwired: 5 out]
            n65 = call-poly <vilib>:"Stop Motion.flx"("Stop Type (Decel)"=w192, "error in (no error)"=w193, "Axis or Vector Space"=w186, "Board ID"=w194) -> ("error out"=w189:errorcluster, "Resource Output"=w190:T13, "Bd ID Out"=w191:T9)  [unwired: 1 in, 2 out]
            n66 = call <vilib>:"Read Position.flx"("error in (no error)"=w189, "Axis"=w190, "Board ID"=w191) -> ("error out"=w185:errorcluster, "Position"=w188:i32)  [unwired: 5 out]
            n67 = Divide(x=w188, y=w184) -> (x/y=w187:dbl)
            n68 = local write "X Position (mm)"(w187) -> ()
          }
          event "Ax2Plus": Mouse Up; "Ax2Plus": Mouse Leave {
            n69 = event-data() -> ()  [unwired: 5 out]
            n70 = call-poly <vilib>:"Stop Motion.flx"("Stop Type (Decel)"=w202, "error in (no error)"=w199, "Axis or Vector Space"=w200, "Board ID"=w201) -> ("error out"=w204:errorcluster, "Resource Output"=w205:T13, "Bd ID Out"=w206:T9)  [unwired: 1 in, 2 out]
            n71 = call <vilib>:"Read Position.flx"("error in (no error)"=w204, "Axis"=w205, "Board ID"=w206) -> ("error out"=w197:errorcluster, "Position"=w203:i32)  [unwired: 5 out]
            n72 = Divide(x=w203, y=w196) -> (x/y=w198:dbl)
            n73 = local write "Y Position (mm)"(w198) -> ()
          }
          event "Ax3Plus": Mouse Up; "Ax3Plus": Mouse Leave {
            n74 = event-data() -> ()  [unwired: 5 out]
            n75 = call-poly <vilib>:"Stop Motion.flx"("Stop Type (Decel)"=w216, "error in (no error)"=w213, "Axis or Vector Space"=w214, "Board ID"=w215) -> ("error out"=w219:errorcluster, "Resource Output"=w218:T13, "Bd ID Out"=w217:T9)  [unwired: 1 in, 2 out]
            n76 = call <vilib>:"Read Position.flx"("error in (no error)"=w219, "Axis"=w218, "Board ID"=w217) -> ("error out"=w212:errorcluster, "Position"=w220:i32)  [unwired: 5 out]
            n77 = Divide(x=w220, y=w208) -> (x/y=w211:dbl)
            n78 = Multiply(x=w211, y=w209) -> (x*y=w210:dbl)
            n79 = local write "Z Position (mm)"(w210) -> ()
          }
          event "Ax4Plus": Mouse Up; "Ax4Plus": Mouse Leave {
            n80 = event-data() -> ()  [unwired: 5 out]
            n81 = call-poly <vilib>:"Stop Motion.flx"("Stop Type (Decel)"=w232, "error in (no error)"=w229, "Axis or Vector Space"=w230, "Board ID"=w231) -> ("error out"=w226:errorcluster, "Resource Output"=w227:T13, "Bd ID Out"=w228:T9)  [unwired: 1 in, 2 out]
            n82 = case shown="\"NI 735x\", Default" w224 {
              tunnel: w228 -> [w238 w243]
              tunnel: w227 -> [w237 w242]
              tunnel: w226 -> [w236 w244]
              tunnel: [w235 w241] -> w223
              tunnel: [w234 w240] -> w225
              tunnel: w222 -> [w233 _]
              frame "NI 735x", Default {
                n83 = call <vilib>:"Read Position.flx"("error in (no error)"=w236, "Axis"=w237, "Board ID"=w238) -> ("error out"=w235:errorcluster, "Position"=w239:i32)  [unwired: 5 out]
                n84 = Divide(x=w239, y=w233) -> (x/y=w234:dbl)
              }
              frame "No Motion Card" {
                n85 = call <vilib>:"Read Position.flx"("error in (no error)"=w244, "Axis"=w242, "Board ID"=w243) -> ("error out"=w241:errorcluster, "Position"=w246:i32)  [unwired: 5 out]
                n86 = Divide(x=w246, y=4000) -> (x/y=w247:dbl)
                n87 = Multiply(x=360.0, y=w247) -> (x*y=w249:dbl)
                n88 = Quotient & Remainder(x=w249, y=360.0) -> (x-y*floor(x/y)=w240:dbl)  [unwired: 1 out]
              }
            }
            n89 = local write "W Position (mm)"(w225) -> ()
          }
          event "Ax1Minus": Mouse Down? {
            n90 = event-data() -> ()  [unwired: 2 out]
            n91 = Negate(x=w253) -> (-x=w252:i32)
            n92 = call <vilib>:"Load Target Position.flx"("Target Position (0)"=w252, "error in (no error)"=w258, "Axis"=w259, "Board ID"=w260) -> ("error out"=w257:errorcluster, "Resource Output"=w256:T13, "Bd ID Out"=w255:T9)  [unwired: 3 out]
            n93 = call-poly <vilib>:"Start Motion.flx"("error in (no error)"=w257, "Axis or Vector Space"=w256, "Board ID"=w255) -> ("error out"=w254:errorcluster)  [unwired: 1 in, 4 out]
            n94 = event-data() -> ()  [unwired: 1 in, 2 out]
          }
          event "Ax2Minus": Mouse Down? {
            n95 = event-data() -> ()  [unwired: 2 out]
            n96 = Negate(x=w263) -> (-x=w262:i32)
            n97 = call <vilib>:"Load Target Position.flx"("Target Position (0)"=w262, "error in (no error)"=w265, "Axis"=w266, "Board ID"=w267) -> ("error out"=w270:errorcluster, "Resource Output"=w269:T13, "Bd ID Out"=w268:T9)  [unwired: 3 out]
            n98 = call-poly <vilib>:"Start Motion.flx"("error in (no error)"=w270, "Axis or Vector Space"=w269, "Board ID"=w268) -> ("error out"=w264:errorcluster)  [unwired: 1 in, 4 out]
            n99 = event-data() -> ()  [unwired: 1 in, 5 out]
          }
          event "Ax3Minus": Mouse Down? {
            n100 = event-data() -> ()  [unwired: 2 out]
            n101 = Negate(x=w272) -> (-x=w274:i32)
            n102 = Multiply(x=w274, y=w276) -> (x*y=w275:i32)
            n103 = call <vilib>:"Load Target Position.flx"("Target Position (0)"=w275, "error in (no error)"=w277, "Axis"=w278, "Board ID"=w279) -> ("error out"=w282:errorcluster, "Resource Output"=w281:T13, "Bd ID Out"=w280:T9)  [unwired: 3 out]
            n104 = call-poly <vilib>:"Start Motion.flx"("error in (no error)"=w282, "Axis or Vector Space"=w281, "Board ID"=w280) -> ("error out"=w273:errorcluster)  [unwired: 1 in, 4 out]
            n105 = event-data() -> ()  [unwired: 1 in, 5 out]
          }
          event "Ax4Minus": Mouse Down? {
            n106 = event-data() -> ()  [unwired: 2 out]
            n107 = Negate(x=w285) -> (-x=w284:i32)
            n108 = call <vilib>:"Load Target Position.flx"("Target Position (0)"=w284, "error in (no error)"=w287, "Axis"=w288, "Board ID"=w289) -> ("error out"=w290:errorcluster, "Resource Output"=w291:T13, "Bd ID Out"=w292:T9)  [unwired: 3 out]
            n109 = call-poly <vilib>:"Start Motion.flx"("error in (no error)"=w290, "Axis or Vector Space"=w291, "Board ID"=w292) -> ("error out"=w286:errorcluster)  [unwired: 1 in, 4 out]
            n110 = event-data() -> ()  [unwired: 1 in, 5 out]
          }
          event "Ax1Minus": Mouse Up; "Ax1Minus": Mouse Leave {
            n111 = event-data() -> ()  [unwired: 5 out]
            n112 = call-poly <vilib>:"Stop Motion.flx"("Stop Type (Decel)"=w304, "error in (no error)"=w302, "Axis or Vector Space"=w295, "Board ID"=w303) -> ("error out"=w299:errorcluster, "Resource Output"=w300:T13, "Bd ID Out"=w301:T9)  [unwired: 1 in, 2 out]
            n113 = call <vilib>:"Read Position.flx"("error in (no error)"=w299, "Axis"=w300, "Board ID"=w301) -> ("error out"=w296:errorcluster, "Position"=w298:i32)  [unwired: 5 out]
            n114 = Divide(x=w298, y=w294) -> (x/y=w297:dbl)
            n115 = local write "X Position (mm)"(w297) -> ()
          }
          event "Ax2Minus": Mouse Up; "Ax2Minus": Mouse Leave {
            n116 = event-data() -> ()  [unwired: 5 out]
            n117 = call-poly <vilib>:"Stop Motion.flx"("Stop Type (Decel)"=w312, "error in (no error)"=w309, "Axis or Vector Space"=w310, "Board ID"=w311) -> ("error out"=w315:errorcluster, "Resource Output"=w314:T13, "Bd ID Out"=w313:T9)  [unwired: 1 in, 2 out]
            n118 = call <vilib>:"Read Position.flx"("error in (no error)"=w315, "Axis"=w314, "Board ID"=w313) -> ("error out"=w307:errorcluster, "Position"=w316:i32)  [unwired: 5 out]
            n119 = Divide(x=w316, y=w306) -> (x/y=w308:dbl)
            n120 = local write "Y Position (mm)"(w308) -> ()
          }
          event "Ax3Minus": Mouse Up; "Ax3Minus": Mouse Leave {
            n121 = event-data() -> ()  [unwired: 5 out]
            n122 = call-poly <vilib>:"Stop Motion.flx"("Stop Type (Decel)"=w326, "error in (no error)"=w323, "Axis or Vector Space"=w324, "Board ID"=w325) -> ("error out"=w329:errorcluster, "Resource Output"=w328:T13, "Bd ID Out"=w327:T9)  [unwired: 1 in, 2 out]
            n123 = call <vilib>:"Read Position.flx"("error in (no error)"=w329, "Axis"=w328, "Board ID"=w327) -> ("error out"=w322:errorcluster, "Position"=w330:i32)  [unwired: 5 out]
            n124 = Divide(x=w330, y=w318) -> (x/y=w321:dbl)
            n125 = Multiply(x=w321, y=w319) -> (x*y=w320:dbl)
            n126 = local write "Z Position (mm)"(w320) -> ()
          }
          event "Ax4Minus": Mouse Up; "Ax4Minus": Mouse Leave {
            n127 = event-data() -> ()  [unwired: 5 out]
            n128 = call-poly <vilib>:"Stop Motion.flx"("Stop Type (Decel)"=w339, "error in (no error)"=w336, "Axis or Vector Space"=w337, "Board ID"=w338) -> ("error out"=w340:errorcluster, "Resource Output"=w341:T13, "Bd ID Out"=w342:T9)  [unwired: 1 in, 2 out]
            n129 = case shown="\"NI 735x\", Default" w334 {
              tunnel: w342 -> [w353 w359]
              tunnel: w341 -> [w352 w358]
              tunnel: w340 -> [w351 w357]
              tunnel: [w346 w356] -> w333
              tunnel: [w343 w355] -> w335
              tunnel: w332 -> [_ w354]
              frame "No Motion Card" {
                n130 = call <vilib>:"Read Position.flx"("error in (no error)"=w351, "Axis"=w352, "Board ID"=w353) -> ("error out"=w346:errorcluster, "Position"=w349:i32)  [unwired: 5 out]
                n131 = Divide(x=w349, y=4000) -> (x/y=w348:dbl)
                n132 = Multiply(x=360.0, y=w348) -> (x*y=w344:dbl)
                n133 = Quotient & Remainder(x=w344, y=360.0) -> (x-y*floor(x/y)=w343:dbl)  [unwired: 1 out]
              }
              frame "NI 735x", Default {
                n134 = call <vilib>:"Read Position.flx"("error in (no error)"=w357, "Axis"=w358, "Board ID"=w359) -> ("error out"=w356:errorcluster, "Position"=w360:i32)  [unwired: 5 out]
                n135 = Divide(x=w360, y=w354) -> (x/y=w355:dbl)
              }
            }
            n136 = local write "W Position (mm)"(w335) -> ()
          }
          event "Rst1": Value Change {
            w363 = 0 ("Primary Reset Position (0)")
            n137 = event-data() -> ()  [unwired: 3 out]
            n138 = call <vilib>:"Reset Position.flx"("Primary Reset Position (0)"=w363, "error in (no error)"=w365, "Axis"=w364, "Board ID"=w366) -> ("error out"=w362:errorcluster)  [unwired: 1 in, 4 out]
            n139 = local write "X Position (mm)"(w363) -> ()
          }
          event "Rst2": Value Change {
            w369 = 0 ("Primary Reset Position (0)")
            n140 = event-data() -> ()  [unwired: 4 out]
            n141 = call <vilib>:"Reset Position.flx"("Primary Reset Position (0)"=w369, "error in (no error)"=w370, "Axis"=w371, "Board ID"=w372) -> ("error out"=w368:errorcluster)  [unwired: 1 in, 4 out]
            n142 = local write "Y Position (mm)"(w369) -> ()
          }
          event "Rst3": Value Change {
            w375 = 0 ("Primary Reset Position (0)")
            n143 = event-data() -> ()  [unwired: 4 out]
            n144 = call <vilib>:"Reset Position.flx"("Primary Reset Position (0)"=w375, "error in (no error)"=w376, "Axis"=w377, "Board ID"=w378) -> ("error out"=w374:errorcluster)  [unwired: 1 in, 4 out]
            n145 = local write "Z Position (mm)"(w375) -> ()
          }
          event "Rst4": Value Change {
            w380 = 0 ("Primary Reset Position (0)")
            n146 = event-data() -> ()  [unwired: 3 out]
            n147 = call <vilib>:"Reset Position.flx"("Primary Reset Position (0)"=w380, "error in (no error)"=w382, "Axis"=w383, "Board ID"=w384) -> ("error out"=w381:errorcluster)  [unwired: 1 in, 4 out]
            n148 = local write "W Position (mm)"(w380) -> ()
          }
          event "FinePl1": Value Change {
            # "# of counts for 1cm"
            n149 = event-data() -> ()  [unwired: 2 out]
            n150 = expression code="x*10"(w386) -> (w387:i32)
            n151 = call <vilib>:"Load Target Position.flx"("Target Position (0)"=w387, "error in (no error)"=w390, "Axis"=w388, "Board ID"=w391) -> ("error out"=w393:errorcluster, "Resource Output"=w392:T13, "Bd ID Out"=w394:T9)  [unwired: 3 out]
            n152 = call-poly <vilib>:"Start Motion.flx"("error in (no error)"=w393, "Axis or Vector Space"=w392, "Board ID"=w394) -> ("error out"=w389:errorcluster)  [unwired: 1 in, 4 out]
          }
          event "FinePl2": Value Change {
            # "# of counts for 1cm"
            n153 = event-data() -> ()  [unwired: 2 out]
            n154 = expression code="x*10"(w397) -> (w396:i32)
            n155 = call <vilib>:"Load Target Position.flx"("Target Position (0)"=w396, "error in (no error)"=w399, "Axis"=w400, "Board ID"=w401) -> ("error out"=w403:errorcluster, "Resource Output"=w402:T13, "Bd ID Out"=w404:T9)  [unwired: 3 out]
            n156 = call-poly <vilib>:"Start Motion.flx"("error in (no error)"=w403, "Axis or Vector Space"=w402, "Board ID"=w404) -> ("error out"=w398:errorcluster)  [unwired: 1 in, 4 out]
          }
          event "FinePl3": Value Change {
            # "# of counts for 1cm"
            n157 = event-data() -> ()  [unwired: 2 out]
            n158 = expression code="x*10"(w407) -> (w406:i32)
            n159 = Multiply(x=w406, y=w410) -> (x*y=w409:i32)
            n160 = call <vilib>:"Load Target Position.flx"("Target Position (0)"=w409, "error in (no error)"=w411, "Axis"=w412, "Board ID"=w413) -> ("error out"=w415:errorcluster, "Resource Output"=w414:T13, "Bd ID Out"=w416:T9)  [unwired: 3 out]
            n161 = call-poly <vilib>:"Start Motion.flx"("error in (no error)"=w415, "Axis or Vector Space"=w414, "Board ID"=w416) -> ("error out"=w408:errorcluster)  [unwired: 1 in, 4 out]
          }
          event "FinePl4": Value Change {
            n162 = event-data() -> ()  [unwired: 2 out]
            n163 = expression code="x*10"(w419) -> (w418:i32)
            n164 = case shown="\"Newport ESP\"" w420 {
              tunnel: w424 -> [w429 w436]
              tunnel: w423 -> [w428 w435]
              tunnel: w422 -> [w427 w434]
              tunnel: [w426 w433] -> w421
              tunnel: w418 -> [w425 _]
              frame "NI 735x", Default {
                (unwired) 10000 ("x")
                # "# of counts for 1cm"
                n165 = call <vilib>:"Load Target Position.flx"("Target Position (0)"=w425, "error in (no error)"=w427, "Axis"=w428, "Board ID"=w429) -> ("error out"=w431:errorcluster, "Resource Output"=w430:T13, "Bd ID Out"=w432:T9)  [unwired: 3 out]
                n166 = call-poly <vilib>:"Start Motion.flx"("error in (no error)"=w431, "Axis or Vector Space"=w430, "Board ID"=w432) -> ("error out"=w426:errorcluster)  [unwired: 1 in, 4 out]
              }
              frame "Newport ESP" {
                # "# of counts for 1 revolution"
                n167 = call <vilib>:"Load Target Position.flx"("Target Position (0)"=4000 ("x"), "error in (no error)"=w434, "Axis"=w435, "Board ID"=w436) -> ("error out"=w439:errorcluster, "Resource Output"=w438:T13, "Bd ID Out"=w440:T9)  [unwired: 3 out]
                n168 = call-poly <vilib>:"Start Motion.flx"("error in (no error)"=w439, "Axis or Vector Space"=w438, "Board ID"=w440) -> ("error out"=w433:errorcluster)  [unwired: 1 in, 4 out]
              }
            }
          }
          event "FineMi1": Value Change {
            # "# of counts for 1cm"
            n169 = event-data() -> ()  [unwired: 4 out]
            n170 = expression code="x*-10"(w442) -> (w443:i32)
            n171 = call <vilib>:"Load Target Position.flx"("Target Position (0)"=w443, "error in (no error)"=w446, "Axis"=w444, "Board ID"=w447) -> ("error out"=w449:errorcluster, "Resource Output"=w450:T13, "Bd ID Out"=w448:T9)  [unwired: 3 out]
            n172 = call-poly <vilib>:"Start Motion.flx"("error in (no error)"=w449, "Axis or Vector Space"=w450, "Board ID"=w448) -> ("error out"=w445:errorcluster)  [unwired: 1 in, 4 out]
          }
          event "FineMi2": Value Change {
            # "# of counts for 1cm"
            n173 = event-data() -> ()  [unwired: 4 out]
            n174 = expression code="x*-10"(w453) -> (w452:i32)
            n175 = call <vilib>:"Load Target Position.flx"("Target Position (0)"=w452, "error in (no error)"=w455, "Axis"=w456, "Board ID"=w457) -> ("error out"=w459:errorcluster, "Resource Output"=w460:T13, "Bd ID Out"=w458:T9)  [unwired: 3 out]
            n176 = call-poly <vilib>:"Start Motion.flx"("error in (no error)"=w459, "Axis or Vector Space"=w460, "Board ID"=w458) -> ("error out"=w454:errorcluster)  [unwired: 1 in, 4 out]
          }
          event "FineMi3": Value Change {
            # "# of counts for 1cm"
            n177 = event-data() -> ()  [unwired: 2 out]
            n178 = expression code="x*-10"(w463) -> (w462:i32)
            n179 = Multiply(x=w462, y=w466) -> (x*y=w465:i32)
            n180 = call <vilib>:"Load Target Position.flx"("Target Position (0)"=w465, "error in (no error)"=w467, "Axis"=w468, "Board ID"=w469) -> ("error out"=w471:errorcluster, "Resource Output"=w472:T13, "Bd ID Out"=w470:T9)  [unwired: 3 out]
            n181 = call-poly <vilib>:"Start Motion.flx"("error in (no error)"=w471, "Axis or Vector Space"=w472, "Board ID"=w470) -> ("error out"=w464:errorcluster)  [unwired: 1 in, 4 out]
          }
          event "FineMi4": Value Change {
            n182 = event-data() -> ()  [unwired: 2 out]
            n183 = expression code="x*-10"(w475) -> (w474:i32)
            n184 = case shown="\"NI 735x\", Default" w476 {
              tunnel: w480 -> [w485 w492]
              tunnel: w479 -> [w484 w491]
              tunnel: w478 -> [w483 w490]
              tunnel: [w482 w489] -> w477
              tunnel: w474 -> [w481 _]
              frame "NI 735x", Default {
                # "# of counts for 1cm"
                n185 = call <vilib>:"Load Target Position.flx"("Target Position (0)"=w481, "error in (no error)"=w483, "Axis"=w484, "Board ID"=w485) -> ("error out"=w487:errorcluster, "Resource Output"=w488:T13, "Bd ID Out"=w486:T9)  [unwired: 3 out]
                n186 = call-poly <vilib>:"Start Motion.flx"("error in (no error)"=w487, "Axis or Vector Space"=w488, "Board ID"=w486) -> ("error out"=w482:errorcluster)  [unwired: 1 in, 4 out]
              }
              frame "No Motion Card" {
                # "# of counts for 1 revolution"
                n187 = call <vilib>:"Load Target Position.flx"("Target Position (0)"=-4000 ("x"), "error in (no error)"=w490, "Axis"=w491, "Board ID"=w492) -> ("error out"=w494:errorcluster, "Resource Output"=w495:T13, "Bd ID Out"=w493:T9)  [unwired: 3 out]
                n188 = call-poly <vilib>:"Start Motion.flx"("error in (no error)"=w494, "Axis or Vector Space"=w495, "Board ID"=w493) -> ("error out"=w489:errorcluster)  [unwired: 1 in, 4 out]
              }
            }
          }
          event "X Position (mm)": Value Change {
            n189 = event-data() -> ("NewVal"=w501:dbl)  [unwired: 1 out]
            n190 = call <vilib>:"Read Position.flx"("error in (no error)"=w512, "Axis"=w499, "Board ID"=w513) -> ("error out"=w509:errorcluster, "Resource Output"=w510:T13, "Bd ID Out"=w511:T9, "Position"=w508:i32)  [unwired: 3 out]
            n191 = Multiply(x=w501, y=w498) -> (x*y=w507:dbl)
            n192 = Subtract(x=w507, y=w508) -> (x-y=w506:dbl)
            n193 = To Long Integer(number=w506) -> (32bit integer=w505:i32)
            n194 = call <vilib>:"Load Target Position.flx"("Target Position (0)"=w505, "error in (no error)"=w509, "Axis"=w510, "Board ID"=w511) -> ("error out"=w502:errorcluster, "Resource Output"=w503:T13, "Bd ID Out"=w504:T9)  [unwired: 3 out]
            n195 = call-poly <vilib>:"Start Motion.flx"("error in (no error)"=w502, "Axis or Vector Space"=w503, "Board ID"=w504) -> ("error out"=w500:errorcluster)  [unwired: 1 in, 4 out]
          }
          event "Y Position (mm)": Value Change {
            n196 = event-data() -> ("NewVal"=w517:dbl)  [unwired: 1 out]
            n197 = call <vilib>:"Read Position.flx"("error in (no error)"=w519, "Axis"=w518, "Board ID"=w520) -> ("error out"=w528:errorcluster, "Resource Output"=w529:T13, "Bd ID Out"=w530:T9, "Position"=w527:i32)  [unwired: 3 out]
            n198 = Multiply(x=w517, y=w515) -> (x*y=w526:dbl)
            n199 = Subtract(x=w526, y=w527) -> (x-y=w525:dbl)
            n200 = To Long Integer(number=w525) -> (32bit integer=w524:i32)
            n201 = call <vilib>:"Load Target Position.flx"("Target Position (0)"=w524, "error in (no error)"=w528, "Axis"=w529, "Board ID"=w530) -> ("error out"=w521:errorcluster, "Resource Output"=w522:T13, "Bd ID Out"=w523:T9)  [unwired: 3 out]
            n202 = call-poly <vilib>:"Start Motion.flx"("error in (no error)"=w521, "Axis or Vector Space"=w522, "Board ID"=w523) -> ("error out"=w516:errorcluster)  [unwired: 1 in, 4 out]
          }
          event "Z Position (mm)": Value Change {
            n203 = event-data() -> ("NewVal"=w535:dbl)  [unwired: 1 out]
            n204 = call <vilib>:"Read Position.flx"("error in (no error)"=w536, "Axis"=w537, "Board ID"=w538) -> ("error out"=w546:errorcluster, "Resource Output"=w547:T13, "Bd ID Out"=w548:T9, "Position"=w545:i32)  [unwired: 3 out]
            n205 = Compound Arithmetic op=MULTIPLY(w535, w532, w533) -> (w544:dbl)
            n206 = Subtract(x=w544, y=w545) -> (x-y=w543:dbl)
            n207 = To Long Integer(number=w543) -> (32bit integer=w542:i32)
            n208 = call <vilib>:"Load Target Position.flx"("Target Position (0)"=w542, "error in (no error)"=w546, "Axis"=w547, "Board ID"=w548) -> ("error out"=w539:errorcluster, "Resource Output"=w540:T13, "Bd ID Out"=w541:T9)  [unwired: 3 out]
            n209 = call-poly <vilib>:"Start Motion.flx"("error in (no error)"=w539, "Axis or Vector Space"=w540, "Board ID"=w541) -> ("error out"=w534:errorcluster)  [unwired: 1 in, 4 out]
          }
          event "W Position (mm)": Value Change {
            n210 = event-data() -> ("NewVal"=w553:dbl)  [unwired: 1 out]
            n211 = call <vilib>:"Read Position.flx"("error in (no error)"=w555, "Axis"=w556, "Board ID"=w557) -> ("error out"=w562:errorcluster, "Resource Output"=w563:T13, "Bd ID Out"=w564:T9, "Position"=w554:i32)  [unwired: 3 out]
            n212 = case shown="\"NI 735x\", Default" w551 {
              tunnel: [w566 w572] -> w561
              tunnel: w554 -> [w567 w578]
              tunnel: w553 -> [w568 w573]
              tunnel: w550 -> [w565 _]
              frame "NI 735x", Default {
                n213 = Multiply(x=w568, y=w565) -> (x*y=w569:dbl)
                n214 = Subtract(x=w569, y=w567) -> (x-y=w566:dbl)
              }
              frame "No Motion Card" {
                w571 = 360.0 ("y")
                w570 = 4000 ("y")
                n215 = Divide(x=w578, y=w570) -> (x/y=w577:dbl)
                n216 = Multiply(x=w577, y=w571) -> (x*y=w576:dbl)
                n217 = Quotient & Remainder(x=w573, y=w571) -> (x-y*floor(x/y)=w579:dbl)  [unwired: 1 out]
                n218 = Divide(x=w579, y=w571) -> (x/y=w580:dbl)
                n219 = Quotient & Remainder(x=w576, y=w571) -> (x-y*floor(x/y)=w575:dbl)  [unwired: 1 out]
                n220 = Multiply(x=w575, y=w570) -> (x*y=w574:dbl)
                n221 = Multiply(x=w580, y=w570) -> (x*y=w581:dbl)
                n222 = Subtract(x=w581, y=w574) -> (x-y=w572:dbl)
              }
            }
            n223 = call <vilib>:"Load Target Position.flx"("Target Position (0)"=w561, "error in (no error)"=w562, "Axis"=w563, "Board ID"=w564) -> ("error out"=w558:errorcluster, "Resource Output"=w559:T13, "Bd ID Out"=w560:T9)  [unwired: 3 out]
            n224 = call-poly <vilib>:"Start Motion.flx"("error in (no error)"=w558, "Axis or Vector Space"=w559, "Board ID"=w560) -> ("error out"=w552:errorcluster)  [unwired: 1 in, 4 out]
          }
          event "Select V&A": Value Change {
            n225 = event-data() -> ()  [unwired: 7 out]
            n226 = call "UpdateVandAGlobals.vi"("Motion Settings"=w583) -> ("Motion Settings Out"=w582:T1)  [unwired: 3 in, 1 out]
            n227 = Unbundle By Name(w582) -> ("Motor Parameters.velocity ct/s"=w585:dbl[], "Motor Parameters.accel ct/s^2"=w587:dbl[])
            n228 = for {
              tunnel: w589 -> [w597]
              tunnel: [w592] -> w586
              tunnel: w588 -> [w596]
              tunnel: w587 -> [w595] mode=indexing
              tunnel: w585 -> [w590] mode=indexing
              i -> [w599]
              n229 = Increment(x=w599) -> (x+1=w598:i32)
              n230 = call "Load Acceleration/Deceleration.flx"("Acceleration (100000)"=w595, "error in (no error)"=w597, "Axis or Vector Space"=w598, "Board ID"=w596) -> ("error out"=w593:errorcluster, "Resource Output"=w591:T13, "Bd ID Out"=w594:T9)  [unwired: 1 in, 2 out]
              n231 = call <vilib>:"Load Velocity.flx"("Velocity (10000)"=w590, "error in (no error)"=w593, "Axis or Vector Space"=w591, "Board ID"=w594) -> ("error out"=w592:errorcluster)  [unwired: 5 out]
            }
            n232 = local write "Select V&A"(FALSE ("Select V&A")) -> ()
          }
          event Key Down {
            w607 = T14[] [enum."Up", enum."Down", enum."Left", enum."Right", enum."PageUp", enum."PageDown"] items=["ASCII", "Enter", "Return", "Shift", "Ctrl", "Alt", "Cmd", "Opt", "Caps", "NumLock", "Clear", "Break", "Up", "Down", "Left", "Right", "Insert", "Delete", "Home", "End", "PageUp", "PageDown", "Escape", "Help", "Pause", "ScrollLock", "F1", "F2", "F3", "F4", "F5", "F6", "F7", "F8", "F9", "F10", "F11", "F12", "F13", "F14", "F15", "F16", "F17", "F18", "F19", "F20", "F21", "F22", "F23", "F24", "Play", "VolumeUp", "VolumeDown", "Mute", "Two Byte Char"]
            n233 = event-data() -> ("VKey"=w609:T14, "Char"=w613:i16, "PlatMods"=w616:T15)  [unwired: 1 out]
            n234 = property on="Y Position (mm)" class="DigNum (strict)"() -> ("Key Focus"=w606:bool)  [unwired: 2 in, 2 out]
            n235 = property on="W Position (mm)" class="DigNum (strict)"() -> ("Key Focus"=w605:bool)  [unwired: 2 in, 2 out]
            n236 = property on="Z Position (mm)" class="DigNum (strict)"() -> ("Key Focus"=w604:bool)  [unwired: 2 in, 2 out]
            n237 = property on="X Position (mm)" class="DigNum (strict)"() -> ("Key Focus"=w603:bool)  [unwired: 2 in, 2 out]
            n238 = property on="Inc. Step\nSize (mm)" class="DigNum (strict)"() -> ("Key Focus"=w602:bool)  [unwired: 2 in, 2 out]
            n239 = Equal?(x=w613, y=i16[] [90, 122, 67, 99]) -> (x = y?=w611:bool[])
            n240 = Equal?(x=w609, y=w607) -> (x = y?=w614:bool[])
            n241 = Or Array Elements(Boolean array=w611) -> (logical OR=w610:bool)
            n242 = Or Array Elements(Boolean array=w614) -> (logical OR=w608:bool)
            n243 = Or(x=w610, y=w608) -> (x .or. y?=w601:bool)
            n244 = Compound Arithmetic op=OR(w606, w605, w604, w603, w602) -> (w600:bool)
            n245 = stacked-sequence {
              tunnel: "Axis Tune" -> [w620 _ _]
              tunnel: w617 -> [_ w632 _]
              tunnel: w616 -> [_ w631 _]
              tunnel: w609 -> [_ w630 _]
              tunnel: w613 -> [_ w629 _]
              tunnel: [_ w628 _] -> w615
              tunnel: w601 -> [w619 _ w636]
              tunnel: w600 -> [_ w627 _]
              frame #0 {
                n246 = case shown="False" w619 {
                  tunnel: w620 -> [_ w622]
                  frame False {
                  }
                  frame True {
                    n247 = case shown="\"Axis 4\"" w622 {
                      tunnel: [w623 w624 w625 w626] -> w621
                      frame "Axis 1", Default {
                        n248 = property on="X Position (mm)" class="DigNum (strict)"() -> ("Value"=w623:dbl)  [unwired: 2 in, 2 out]
                      }
                      frame "Axis 2" {
                        n249 = property on="Y Position (mm)" class="DigNum (strict)"() -> ("Value"=w624:dbl)  [unwired: 2 in, 2 out]
                      }
                      frame "Axis 3" {
                        n250 = property on="Z Position (mm)" class="DigNum (strict)"() -> ("Value"=w625:dbl)  [unwired: 2 in, 2 out]
                      }
                      frame "Axis 4" {
                        n251 = property on="W Position (mm)" class="DigNum (strict)"() -> ("Value"=w626:dbl)  [unwired: 2 in, 2 out]
                      }
                    }
                    n252 = property on="Position (mm) (Abs)" class="DigNum (strict)"("Value"=w621) -> ()  [unwired: 2 in, 2 out]
                  }
                }
              }
              frame #1 {
                n253 = control-ref of="Axis Tune"() -> (w634:refnum<vi>)
                n254 = control-ref of="Position (mm) (Abs)"() -> (w635:refnum<vi>)
                n255 = call "KeyboardNudge.vi"("Axis Tune Refnum"=w634, "Char"=w629, "Position (mm) Refnum"=w635, "Ignore Key Down"=w627, "VKey"=w630, "PlatMods"=w631, "Inc. Step Size (mm)"="Inc. Step\nSize (mm)", "Motion Settings"=w632) -> ("Quit"=w628:bool)  [unwired: 10 in, 1 out]
              }
              frame #2 {
                n256 = case shown="True" w636 {
                  frame False {
                  }
                  frame True {
                    n257 = property on="Axis Tune" class="RadioBtnsControl (strict)"() -> ("Value"=w637:enum32{"Axis 1", "Axis 2", "Axis 3", "Axis 4"})  [unwired: 2 in, 2 out]
                    n258 = case shown="\"Axis 4\"" w637 {
                      tunnel: "Position (mm) (Abs)" -> [w639 w640 w641 w642]
                      frame "Axis 1", Default {
                        n259 = property on="X Position (mm)" class="DigNum (strict)"("Val(Sgnl)"=w639) -> ()  [unwired: 2 in, 2 out]
                      }
                      frame "Axis 2" {
                        n260 = property on="Y Position (mm)" class="DigNum (strict)"("Val(Sgnl)"=w640) -> ()  [unwired: 2 in, 2 out]
                      }
                      frame "Axis 3" {
                        n261 = property on="Z Position (mm)" class="DigNum (strict)"("Val(Sgnl)"=w641) -> ()  [unwired: 2 in, 2 out]
                      }
                      frame "Axis 4" {
                        n262 = property on="W Position (mm)" class="DigNum (strict)"("Val(Sgnl)"=w642) -> ()  [unwired: 2 in, 2 out]
                      }
                    }
                  }
                }
              }
            }
          }
          event "Cent X": Value Change {
            n263 = event-data() -> ("CtlRef"=w651:refnum<vi>)  [unwired: 1 out]
            n264 = Unbundle By Name(w644) -> ("Motion Profile"=w643:string)
            n265 = Two Button Dialog(message=w648) -> (T button?=w647:bool)  [unwired: 2 in]
            n266 = case shown="True" w647 {
              tunnel: w646 -> [_ w657]
              tunnel: w645 -> [_ w656]
              tunnel: w651 -> [_ w655]
              tunnel: w650 -> [_ w654]
              tunnel: w649 -> [_ w653]
              tunnel: w643 -> [_ w652]
              frame False {
              }
              frame True {
                n267 = case shown="\"XY_Stage\"" w652 {
                  tunnel: w657 -> [w672 w675]
                  tunnel: w656 -> [w671 _]
                  tunnel: w655 -> [w670 _]
                  tunnel: w654 -> [w669 w676]
                  tunnel: w653 -> [w661 _]
                  frame "False", Default {
                    w664 = TRUE
                    n268 = Not(x=w664) -> (.not. x?=w659:bool)
                    n269 = property on="Property Node" class="Bool"(reference=w670, error in=w669, "Blinking"=w664) -> (reference out=w665:refnum<vi>, error out=w668:errorcluster)
                    n270 = property class="Bool (strict)"(reference=w661, "Value"=w659) -> (reference out=w660:refnum<vi>)  [unwired: 1 in, 1 out]
                    n271 = call <vilib>:"Find Reference.flx"("Search Type"=T6."Center", "error in (no error)"=w668, "Axis or Vector Space"=w671, "Board ID"=w672) -> ("error out"=w673:errorcluster, "Axis or Vector Space Output"=w662:T16, "Bd ID Out"=w663:T9)  [unwired: 5 in]
                    n272 = call <vilib>:"Wait Reference.flx"("error in (no error)"=w673, "Axis or Vector Space"=w662, "Board ID"=w663) -> ("error out"=w667:errorcluster, "Found Reference"=w658:bool)  [unwired: 5 in, 2 out]
                    n273 = property class="Bool (strict)"(reference=w660, "Value"=w658) -> ()  [unwired: 1 in, 2 out]
                    n274 = property on="Property Node" class="Bool"(reference=w665, error in=w667, "Blinking"=FALSE) -> ()  [unwired: 2 out]
                  }
                  frame "XY_Stage" {
                    n275 = disable-structure shown="Disabled" {
                      disable-tunnel: w676 -> [w678 _]
                      disable-tunnel: w675 -> [w677 _]
                      frame Disabled {
                        n276 = call "SetSoftwareLimits.vi"("error in (no error)"=w678, "Board ID"=w677) -> ()  [unwired: 7 in, 3 out]
                      }
                      frame Enabled {
                      }
                    }
                  }
                }
              }
            }
          }
          event "Cent Y": Value Change {
            n277 = event-data() -> ("CtlRef"=w686:refnum<vi>)  [unwired: 1 out]
            n278 = Two Button Dialog(message=w682) -> (T button?=w681:bool)  [unwired: 2 in]
            n279 = Unbundle By Name(w680) -> ("Motion Profile"=w679:string)
            n280 = case shown="True" w681 {
              tunnel: w688 -> [_ w695]
              tunnel: w687 -> [_ w690]
              tunnel: w686 -> [_ w694]
              tunnel: w685 -> [_ w693]
              tunnel: TRUE -> [_ w692]
              tunnel: w683 -> [_ w691]
              tunnel: w679 -> [_ w689]
              frame False {
              }
              frame True {
                n281 = case shown="\"XY_Stage\"" w689 {
                  tunnel: w695 -> [w697 w710]
                  tunnel: w694 -> [_ w707]
                  tunnel: w693 -> [w696 w706]
                  tunnel: w692 -> [_ w703]
                  tunnel: w691 -> [_ w700]
                  tunnel: w690 -> [_ w698]
                  frame "XY_Stage" {
                    n282 = call "SetSoftwareLimits.vi"("error in (no error)"=w696, "Board ID"=w697) -> ()  [unwired: 7 in, 3 out]
                  }
                  frame "True", Default {
                    n283 = Not(x=w703) -> (.not. x?=w701:bool)
                    n284 = property on="Property Node" class="Bool"(reference=w707, error in=w706, "Blinking"=w703) -> (reference out=w708:refnum<vi>, error out=w705:errorcluster)
                    n285 = property class="Bool (strict)"(reference=w700, "Value"=w701) -> (reference out=w699:refnum<vi>)  [unwired: 1 in, 1 out]
                    n286 = call <vilib>:"Find Reference.flx"("Search Type"=T6."Center", "error in (no error)"=w705, "Axis or Vector Space"=w698, "Board ID"=w710) -> ("error out"=w712:errorcluster, "Axis or Vector Space Output"=w711:T16, "Bd ID Out"=w713:T9)  [unwired: 5 in]
                    n287 = call <vilib>:"Wait Reference.flx"("error in (no error)"=w712, "Axis or Vector Space"=w711, "Board ID"=w713) -> ("error out"=w704:errorcluster, "Found Reference"=w702:bool)  [unwired: 5 in, 2 out]
                    n288 = property class="Bool (strict)"(reference=w699, "Value"=w702) -> ()  [unwired: 1 in, 2 out]
                    n289 = property on="Property Node" class="Bool"(reference=w708, error in=w704, "Blinking"=FALSE) -> ()  [unwired: 2 out]
                  }
                }
              }
            }
          }
          event "Cent Z": Value Change {
            n290 = event-data() -> ("CtlRef"=w719:refnum<vi>)  [unwired: 1 out]
            n291 = Two Button Dialog(message=w715) -> (T button?=w716:bool)  [unwired: 2 in]
            n292 = case shown="False" w716 {
              tunnel: w721 -> [_ w735]
              tunnel: w720 -> [_ w734]
              tunnel: w719 -> [_ w731]
              tunnel: w718 -> [_ w730]
              tunnel: w717 -> [_ w726]
              frame False {
              }
              frame True {
                w727 = TRUE
                n293 = property on="Property Node" class="Bool"(reference=w731, error in=w730, "Blinking"=w727) -> (reference out=w732:refnum<vi>, error out=w729:errorcluster)
                n294 = Not(x=w727) -> (.not. x?=w724:bool)
                n295 = call <vilib>:"Find Reference.flx"("Search Type"=T6."Center", "error in (no error)"=w729, "Axis or Vector Space"=w734, "Board ID"=w735) -> ("error out"=w737:errorcluster, "Axis or Vector Space Output"=w736:T16, "Bd ID Out"=w738:T9)  [unwired: 5 in]
                n296 = property class="Bool (strict)"(reference=w726, "Value"=w724) -> (reference out=w725:refnum<vi>)  [unwired: 1 in, 1 out]
                n297 = call <vilib>:"Wait Reference.flx"("error in (no error)"=w737, "Axis or Vector Space"=w736, "Board ID"=w738) -> ("error out"=w728:errorcluster, "Found Reference"=w723:bool)  [unwired: 5 in, 2 out]
                n298 = property on="Property Node" class="Bool"(reference=w732, error in=w728, "Blinking"=FALSE) -> ()  [unwired: 2 out]
                n299 = property class="Bool (strict)"(reference=w725, "Value"=w723) -> ()  [unwired: 1 in, 2 out]
              }
            }
          }
          event "Cent W": Value Change {
            w744 = TRUE
            # "Center the motion stage"
            n300 = event-data() -> ("CtlRef"=w745:refnum<vi>)  [unwired: 2 out]
            n301 = Not(x=w744) -> (.not. x?=w742:bool)
            n302 = property on="Property Node" class="Bool"(reference=w745, error in=w747, "Blinking"=w744) -> (reference out=w749:refnum<vi>, error out=w748:errorcluster)
            n303 = property class="Bool (strict)"(reference=w743, "Value"=w742) -> (reference out=w741:refnum<vi>)  [unwired: 1 in, 1 out]
            n304 = call <vilib>:"Find Reference.flx"("Search Type"=T6."Center", "error in (no error)"=w748, "Axis or Vector Space"=w756, "Board ID"=w757) -> ("error out"=w753:errorcluster, "Axis or Vector Space Output"=w752:T16, "Bd ID Out"=w754:T9)  [unwired: 5 in]
            n305 = call <vilib>:"Wait Reference.flx"("error in (no error)"=w753, "Axis or Vector Space"=w752, "Board ID"=w754) -> ("error out"=w746:errorcluster, "Found Reference"=w740:bool)  [unwired: 5 in, 2 out]
            n306 = property on="Property Node" class="Bool"(reference=w749, error in=w746, "Blinking"=FALSE) -> ()  [unwired: 2 out]
            n307 = property class="Bool (strict)"(reference=w741, "Value"=w740) -> ()  [unwired: 1 in, 2 out]
          }
          event "Cent All": Value Change {
            n308 = event-data() -> ("CtlRef"=w761:refnum<vi>)  [unwired: 1 out]
            n309 = Unbundle By Name(w759) -> ("Motion Profile"=w758:string)
            n310 = case shown="\"XY_Stage\"" w758 {
              tunnel: w763 -> [_ w797]
              tunnel: w762 -> [_ w790]
              tunnel: w761 -> [_ w788]
              tunnel: w760 -> [_ w786]
              tunnel: w759 -> [_ w782]
              frame "XY_Stage" {
              }
              frame "True", Default {
                w787 = TRUE
                # "Center the motion stage"
                n311 = Unbundle By Name(w782) -> ("# Axis"=w781:i8)
                n312 = property on="Property Node" class="Bool"(reference=w788, error in=w790, "Blinking"=w787) -> (reference out=w792:refnum<vi>, error out=w791:errorcluster)
                n313 = Not(x=w787) -> (.not. x?=w785:bool)
                n314 = Cluster To Array(cluster=T7 {"1"=FALSE, "2"=FALSE, "3"=FALSE, "4"=FALSE, "5"=FALSE, "6"=FALSE, "7"=FALSE, "8"=FALSE} ("Axis/VS Map (Disabled)")) -> (array=w767:bool[])
                n315 = property class="Bool (strict)"(reference=w786, "Value"=w785) -> (reference out=w784:refnum<vi>)  [unwired: 1 in, 1 out]
                n316 = Initialize Array(TRUE ("1"), w781) -> (w766:bool[])
                n317 = Insert Into Array(array=w767, index=1, new element=w766) -> (w768:bool[])
                n318 = Array To Cluster(array=w768) -> (cluster=w778:T17)
                n319 = Unbundle(w778) -> ("Axis/VS Map (Disabled)[1]"=w777:bool, "Axis/VS Map (Disabled)[2]"=w770:bool, "Axis/VS Map (Disabled)[3]"=w771:bool, "Axis/VS Map (Disabled)[4]"=w772:bool, "Axis/VS Map (Disabled)[5]"=w773:bool, "Axis/VS Map (Disabled)[6]"=w774:bool, "Axis/VS Map (Disabled)[7]"=w775:bool, "Axis/VS Map (Disabled)[8]"=w776:bool)  [unwired: 1 out]
                n320 = Bundle("Axis/VS Map (Disabled)[1]"=w777, "Axis/VS Map (Disabled)[2]"=w770, "Axis/VS Map (Disabled)[3]"=w771, "Axis/VS Map (Disabled)[4]"=w772, "Axis/VS Map (Disabled)[5]"=w773, "Axis/VS Map (Disabled)[6]"=w774, "Axis/VS Map (Disabled)[7]"=w775, "Axis/VS Map (Disabled)[8]"=w776) -> (w769:T18)  [unwired: 1 in]
                n321 = call <vilib>:"Find Reference.flx"("Search Type"=T6."Center", "Axis/VS Map (Disabled)"=w769, "error in (no error)"=w791, "Board ID"=w797) -> ("error out"=w794:errorcluster, "Bd ID Out"=w795:T9)  [unwired: 5 in, 1 out]
                n322 = call <vilib>:"Wait Reference.flx"("Axis/VS Map (Disabled)"=w769, "error in (no error)"=w794, "Board ID"=w795) -> ("error out"=w789:errorcluster, "Found Reference"=w783:bool)  [unwired: 5 in, 2 out]
                n323 = property on="Property Node" class="Bool"(reference=w792, error in=w789, "Blinking"=FALSE) -> (error out=w764:errorcluster)  [unwired: 1 out]
                n324 = property class="Bool (strict)"(reference=w784, error in=w764, "Value"=w783) -> ()  [unwired: 2 out]
              }
            }
          }
          event "Ratio Num", "Ratio Denom", "Master Axis", "Slave Axis": Value Change {
            n325 = event-data() -> ()  [unwired: 2 out]
            n326 = call <vilib>:"Configure Gear Master.flx"("Master Axis Encoder or ADC"="Master Axis", "Axis"="Slave Axis", "Board ID"=w800) -> ("error out"=w806:errorcluster, "Resource Output"=w805:T13, "Bd ID Out"=w807:T9)  [unwired: 1 in, 2 out]
            n327 = call <vilib>:"Load Gear Ratio.flx"("Ratio Denominator (1)"="Ratio Denom", "Ratio Numerator (0)"="Ratio Num", "Gearing (Absolute)"=TRUE, "error in (no error)"=w806, "Axis"=w805, "Board ID"=w807) -> ()  [unwired: 6 out]
            n328 = Divide(x="Ratio Num", y="Ratio Denom") -> (x/y=w808:dbl)
            n329 = expression code="atan(x)*360/2/3.14159"(w808) -> (→"Angle":dbl)
          }
          event "Enable Gearing": Value Change {
            n330 = event-data() -> ()  [unwired: 2 out]
            n331 = local read "Slave Axis"() -> (w812:u16)
            n332 = call <vilib>:"Enable Gearing Single Axis.flx"("Gearing (Disable)"="Enable Gearing", "Axis"=w812, "Board ID"=w811) -> ()  [unwired: 1 in, 6 out]
          }
          event "Def Abs": Value Change {
            # "Display controls for updating global locations"
            n333 = event-data() -> ("NewVal"=w814:bool)  [unwired: 3 out]
            n334 = case shown="False" w814 {
              tunnel: [T8."Disabled and Grayed Out" ("Disabled") T8."Enabled" ("Disabled")] -> w815
              frame False {
              }
              frame True {
              }
            }
            n335 = property on="Abs X Pos (mm)" class="DigNum (strict)"("DisabledEnum"=w815) -> ()  [unwired: 2 in, 2 out]
            n336 = property on="Abs Y Pos (mm)" class="DigNum (strict)"("DisabledEnum"=w815) -> ()  [unwired: 2 in, 2 out]
            n337 = property on="Abs Z Pos (mm)" class="DigNum (strict)"("DisabledEnum"=w815) -> ()  [unwired: 2 in, 2 out]
            n338 = property on="Abs W Pos (mm)" class="DigNum (strict)"("DisabledEnum"=w815) -> ()  [unwired: 2 in, 2 out]
          }
          event "Abs X Pos (mm)": Value Change {
            # "Update global value and hide indicator.\nNew value will be reflected in position feedback."
            n339 = event-data() -> ()  [unwired: 2 out]
            n340 = Multiply(x=w822, y="Abs X Pos (mm)") -> (x*y=w820:dbl)
            n341 = call <vilib>:"Reset Position.flx"("Primary Reset Position (0)"=w820, "Axis"=w823, "Board ID"=w824) -> ()  [unwired: 2 in, 5 out]
          }
          event "Abs Y Pos (mm)": Value Change {
            # "Update global value and hide indicator.\nNew value will be reflected in position feedback."
            n342 = event-data() -> ()  [unwired: 2 out]
            n343 = Multiply(x=w828, y="Abs Y Pos (mm)") -> (x*y=w827:dbl)
            n344 = call <vilib>:"Reset Position.flx"("Primary Reset Position (0)"=w827, "Axis"=w829, "Board ID"=w830) -> ()  [unwired: 2 in, 5 out]
          }
          event "Abs Z Pos (mm)": Value Change {
            # "Update global value and hide indicator.\nNew value will be reflected in position feedback."
            n345 = event-data() -> ()  [unwired: 2 out]
            n346 = Multiply(x=w836, y="Abs Z Pos (mm)") -> (x*y=w835:dbl)
            n347 = Multiply(x=w835, y=w833) -> (x*y=w834:dbl)
            n348 = call <vilib>:"Reset Position.flx"("Primary Reset Position (0)"=w834, "Axis"=w837, "Board ID"=w838) -> ()  [unwired: 2 in, 5 out]
          }
          event "Abs W Pos (mm)": Value Change {
            # "Update global value and hide indicator.\nNew value will be reflected in position feedback."
            n349 = event-data() -> ()  [unwired: 2 out]
            n350 = Multiply(x=w842, y="Abs W Pos (mm)") -> (x*y=w841:dbl)
            n351 = call <vilib>:"Reset Position.flx"("Primary Reset Position (0)"=w841, "Axis"=w843, "Board ID"=w844) -> ()  [unwired: 2 in, 5 out]
          }
        }
        n352 = Unbundle By Name(w76) -> ("status"=w64:bool)
        n353 = Compound Arithmetic op=OR(w64, "stop", w62) -> (w99:bool)
      }
      "error out" <- w9
      n354 = Unbundle By Name(w4) -> ("Motion Bd ID"=w8:u8)
      n355 = for {
        N: w23 -> [_]
        tunnel: w8 -> [w54]
        tunnel: [w51] -> w26
        tunnel: w9 -> [w50]
        i -> [w53]
        w51 = FALSE ("Gearing (Disable)")
        n356 = Increment(x=w53) -> (x+1=w52:i32)
        n357 = call <vilib>:"Enable Gearing Single Axis.flx"("Gearing (Disable)"=w51, "error in (no error)"=w50, "Axis"=w52, "Board ID"=w54) -> ()  [unwired: 6 out]
      }
      n358 = call "FindLocation.vi"("Motion Settings"=w4) -> ("Motion Settings Out"=→"Motion Settings Out":T1)  [unwired: 2 in, 3 out]
      n359 = local write "Enable Gearing"(w26) -> ()
    }
    frame Enabled {
    }
  }
